vi "运维调试_总磷总氮.vi"() -> ()   [LabVIEW 2016, in "斯坦道总磷总氮.lvlib"]
uses:
  <vilib>/Utility/miscctls.llb/LVPointTypeDef.ctl
  <vilib>/Utility/config.llb/NI_LVConfig.lvlib
  <vilib>/ptbypt/NI_PtbyPt.lvlib
panel:
  in  "总磷参数设置":bool
  in  "总氮参数设置":bool
  in  "模块启用":bool
  in  "串口设置":bool
  in  "备用系数一键写入":bool
  in  "公式一键写入":bool
  in  "流程路径":path=path "C:/Users/std/Documents/斯坦道流程文件/流程.xml"
  in  "曲线模型":cluster{"X^2":dbl, "X":dbl, "B":dbl, "r^2":dbl}(xcontrol)
  out "字符串 2":string
  in  "质控参数设置":bool
  in  "总氮自动测试量程配置":T1
  in  "总磷自动测试量程配置":T1
  out "温度2":sgl
  out "温度1":sgl
  out "ADC":sgl
  out "固件版本号":string
  in  "数组":string[](array[string])
  in  "备用系数写入":bool
  in  "备用系数读取":bool
  in  "备用系数":T2
  in  "量程切换阈值写入":bool
  in  "量程切换阈值读取":bool
  in  "量程切换阈值":cluster{"阈值":dbl, "标液浓度":dbl}
  in  "参数下拉列表":enum16{"总磷", "总氮"}(ring)
  in  "量程下拉列表":enum16{"低量程", "高量程"}(ring)
  in  "测量模式下拉列表":enum16{"水样测量", "零点核查", "跨度核查", "标样核查", "加标回收"}(ring)
  in  "公式":cluster{"X^2":dbl, "X":dbl, "b":dbl}
  in  "写公式":bool
  in  "读公式":bool
  in  "返回":bool
  in  "设置":bool
  out "序列号":string="序列号"
  out "总氮测量数据":T3(xcontrol)
  out "总磷测量数据":T3(xcontrol)
  out "集成报警信息":string
  out "定时启动":bool
  out "总磷总氮运行状态":T4(xcontrol)
  in  "停止":bool
  in  "手动启动":bool
  in  "单步测试":bool
  in  "总磷氨氮调试":u16[](xcontrol)
  out "F3":sgl format="%#.6f"
  out "F2":sgl format="%#.6f"
  out "F1":sgl format="%#.6f"
  out "F0":sgl format="%#.6f"
  out "多列列表框":i32(listbox)
  # "参数设置"
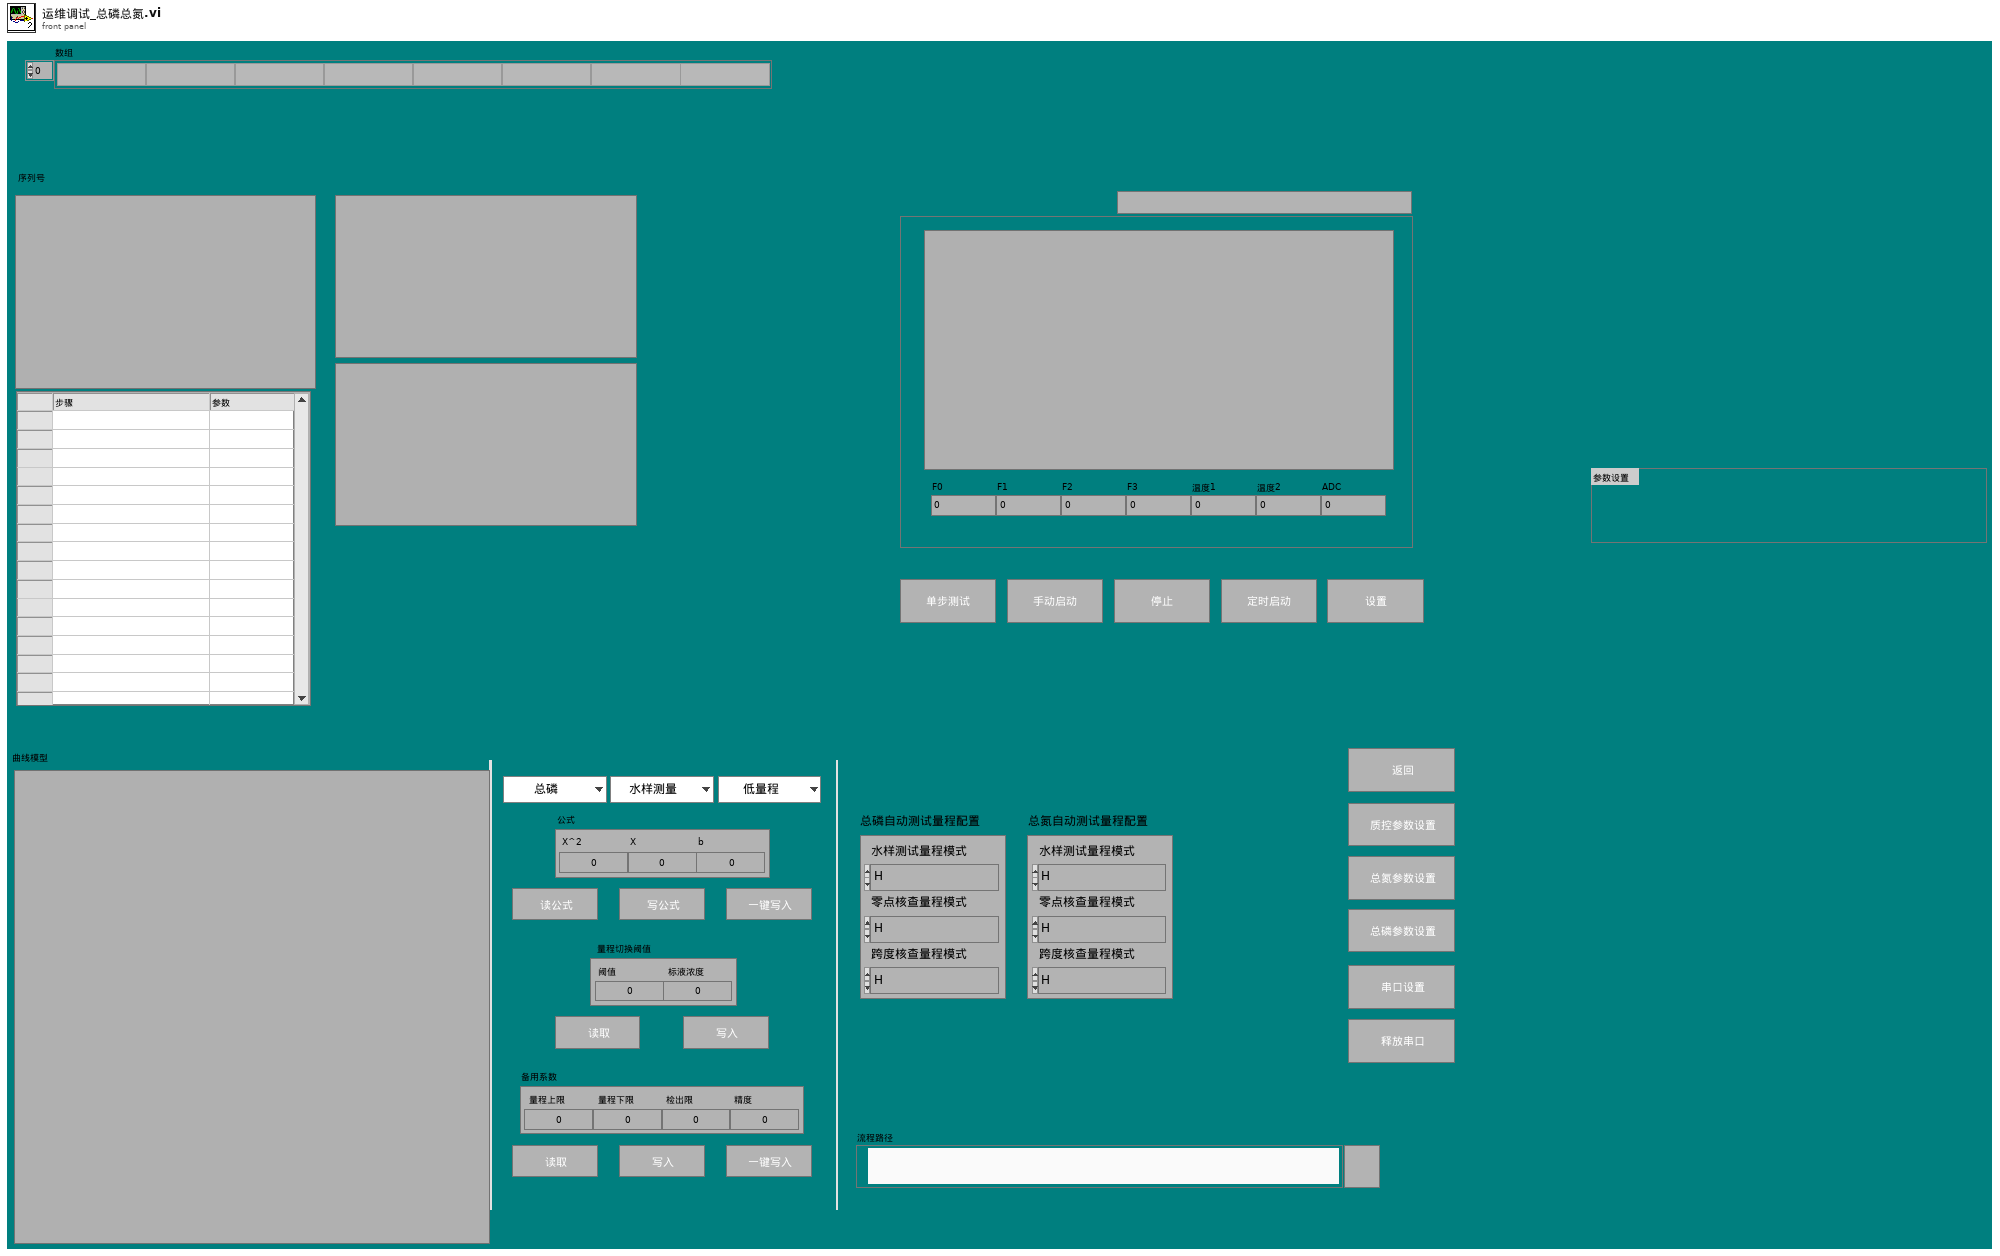
[diagram p1: front panel]
types:
  T1 = cluster{"水样测试量程模式":enum16{"H", "L", "AUTO"}, "空白核查量程模式":enum16{"H", "L", "AUTO"}, "跨度核查量程模式":enum16{"H", "L", "AUTO"}}
  T2 = cluster{"量程上限":dbl, "量程下限":dbl, "检出限":dbl, "精度":dbl}
  T3 = cluster{"flowid":u16, "测量精度":u16, "测量数据区":cluster{"因子编码":u32, "单位":u16, "标样参考值":sgl, "水样数据时间":timestamp, "水样实测值":sgl, "水样数据标识":string, "标样数据时间":timestamp, "标样实测值":sgl, "标样数据标识":string, "空白数据时间":timestamp, "空白实测值":sgl, "空白数据标识":string, "零点核查数据时间":timestamp, "零点核查实测值":sgl, "零点核查数据标识":string, "跨度核查数据时间":timestamp, "跨度核查实测值":sgl, "跨度核查数据标识":string, "加标回收数据时间":timestamp, "加标回收实测值":sgl, "加标回收数据标识":string, "平行样数据时间":timestamp, "平行样实测值":sgl, "平行样数据标识":string, "F0":sgl, "F1":sgl, "F2":sgl, "F3":sgl, "F4":sgl, "F5":sgl, "F6":sgl, "F7":sgl, "温度":sgl, "湿度":sgl, "X值":sgl}}
  T4 = cluster{"系统时间":timestamp, "工作状态":enum16{"空闲", "水样测试", "标样核查", "零点核查", "跨度核查", "空白测试", "平行样测试", "加标回收", "空白校准", "标样校准", "初始化（清洗）"}, "测量模式":enum16{"待机", "连续模式", "周期模式", "定点模式", "受控模式", "手动模式"}, "告警代码":u16, "故障代码":u16, "日志代码":u16, "软件版本":u16, "F0":sgl, "F1":sgl, "F2":sgl, "F3":sgl, "T":sgl, "H":sgl, "id":u16, "flowid":u16, "量程":u16, "总磷控温温度1":sgl, "营养盐控温温度2":sgl, "ADC":sgl}
  T5 = enum16{"启动测量", "标样核查", "零点核查", "跨度核查", "空白测试", "平行样测试", "加标回收", "空白校准", "标样校准", "初始化（清洗）", "停止测试", "仪器重启", "校时", "模式设置", "测量间隔设置"}
  T6 = cluster{"仪器测试类型":enum16{"启动测量", "标样核查", "零点核查", "跨度核查", "空白测试", "平行样测试", "加标回收", "空白校准", "标样校准", "初始化（清洗）", "停止测试", "仪器重启", "校时", "模式设置", "测量间隔设置"}, "周期设置类型":enum16{"定点启动", "间隔启动"}, "定时功能启用":bool, "定时间隔":dbl, "24H周期设置":bool[], "零点核查时间":u16, "跨度核查时间":u16, "质控频次":enum16{"关闭", "每天", "星期一", "星期二", "星期三", "星期四", "星期五", "星期六", "星期日"}}
  T7 = enum16{"关闭", "每天", "星期一", "星期二", "星期三", "星期四", "星期五", "星期六", "星期日"}
  T8 = enum32{"Bad", "Idle", "Run top level", "Running"}
  T9 = typedef "LVDateTimeRec.ctl" = cluster{"秒数的小数部分":dbl, "秒":i32, "分":i32, "时":i32, "日":i32, "月":i32, "年":i32, "天数（周）":i32, "天数（年）":i32, "DST":i32}
  T10 = typedef "LVPointTypeDef.ctl" = cluster{"Horizontal":i16, "Vertical":i16}
  T11 = cluster{"因子编码":u32, "单位":u16, "标样参考值":sgl, "水样数据时间":timestamp, "水样实测值":sgl, "水样数据标识":string, "标样数据时间":timestamp, "标样实测值":sgl, "标样数据标识":string, "空白数据时间":timestamp, "空白实测值":sgl, "空白数据标识":string, "零点核查数据时间":timestamp, "零点核查实测值":sgl, "零点核查数据标识":string, "跨度核查数据时间":timestamp, "跨度核查实测值":sgl, "跨度核查数据标识":string, "加标回收数据时间":timestamp, "加标回收实测值":sgl, "加标回收数据标识":string, "平行样数据时间":timestamp, "平行样实测值":sgl, "平行样数据标识":string, "F0":sgl, "F1":sgl, "F2":sgl, "F3":sgl, "F4":sgl, "F5":sgl, "F6":sgl, "F7":sgl, "温度":sgl, "湿度":sgl, "X值":sgl}
  T12 = enum16{"空闲", "水样测试", "标样核查", "零点核查", "跨度核查", "空白测试", "平行样测试", "加标回收", "空白校准", "标样校准", "初始化（清洗）"}
  T13 = typedef "NI_LVConfig.lvlib/Config Data RefNum.ctl" = refnum<k1>
  T14 = cluster{"启动模式":enum16{"跨度核查", "水样测量", "空白核查", "标样核查", "加标回收"}, "启动参数":u16, "量程":enum16{"低量程", "高量程"}}
  T15 = cluster{"时间标识":timestamp, "设备":string, "日志信息":string, "流程参数":string}
  T16 = cluster{"时间标识":timestamp, "设备":string, "日志信息":string}
  T17 = typedef "LVRowAndColumnUnsignedTypeDef.ctl" = cluster{"Row":u32, "Column":u32}
  T18 = cluster{"参数下拉列表":enum16{"总磷", "总氮"}, "测量模式下拉列表":enum16{"水样测量", "零点核查", "跨度核查", "标样核查", "加标回收"}, "量程下拉列表":enum16{"低量程", "高量程"}}
  T19 = cluster{"站号":u16, "量程切换":enum32{"H", "L", "AUTO"}, "控制命令":enum16{"启动测量", "标样核查", "零点核查", "跨度核查", "空白测试", "平行样测试", "加标回收", "空白校准", "标样校准", "初始化（清洗）", "停止测试", "仪器重启", "校时", "模式设置", "测量间隔设置"}, "模式设置":enum16{"待机", "连续模式", "周期模式", "定点模式", "受控模式", "手动模式"}, "测量间隔":u16}
  T20 = cluster{"总磷跨度值":dbl, "总磷零点标准液浓度":dbl, "总磷跨度标准液浓度":dbl, "总磷标准液标准浓度":dbl, "总氮跨度值":dbl, "总氮零点标准液浓度":dbl, "总氮跨度标准液浓度":dbl, "总氮标准液标准浓度":dbl}
  T21 = cluster{"确定":bool, "总磷跨度值":dbl, "总磷零点标准液浓度":dbl, "总磷跨度标准液浓度":dbl, "总磷标准液标准浓度":dbl, "总氮跨度值":dbl, "总氮零点标准液浓度":dbl, "总氮跨度标准液浓度":dbl, "总氮标准液标准浓度":dbl}
  T22 = cluster{"测量量程":dbl, "测量精度":dbl, "测量间隔":dbl, "消解温度":dbl, "消解时长":dbl, "空白校准时间":timestamp, "曲线截距":dbl, "曲线斜率":dbl, "测量检出限":dbl, "测量信号值":dbl, "线性相关系数":dbl, "二次多项式系数":dbl, "标样校准时间":timestamp, "稀释倍数":dbl, "三项式系数":dbl, "空白标定系数":dbl, "量程系数":dbl, "F0/ORPA":dbl, "F1/ORPB":dbl, "F2/ORPK":dbl, "F3":dbl, "F4":dbl, "F5":dbl, "F6":dbl, "F7":dbl, "X0/滴定数":dbl, "量程":dbl}
  T23 = cluster{"确定":bool, "测量量程":dbl, "测量精度":dbl, "测量间隔":dbl, "消解温度":dbl, "消解时长":dbl, "空白校准时间":timestamp, "曲线截距":dbl, "曲线斜率":dbl, "测量检出限":dbl, "测量信号值":dbl, "线性相关系数":dbl, "二次多项式系数":dbl, "标样校准时间":timestamp, "稀释倍数":dbl, "三项式系数":dbl, "空白标定系数":dbl, "量程系数":dbl, "F0/ORPA":dbl, "F1/ORPB":dbl, "F2/ORPK":dbl, "F3":dbl, "F4":dbl, "F5":dbl, "F6":dbl, "F7":dbl, "X0/滴定数":dbl, "量程":dbl}
  T24 = cluster{"控制命令":enum16{"启动测量", "标样核查", "零点核查", "跨度核查", "空白测试", "平行样测试", "加标回收", "空白校准", "标样校准", "初始化（清洗）", "停止测试", "仪器重启", "校时", "模式设置", "测量间隔设置"}, "周期设置类型":enum16{"定点启动", "间隔启动"}, "定时功能启用":bool, "定时间隔":dbl, "24H周期设置":bool[], "空白核查时间":u16, "跨度核查时间":u16, "质控频次":enum16{"关闭", "每天", "星期一", "星期二", "星期三", "星期四", "星期五", "星期六", "星期日"}}
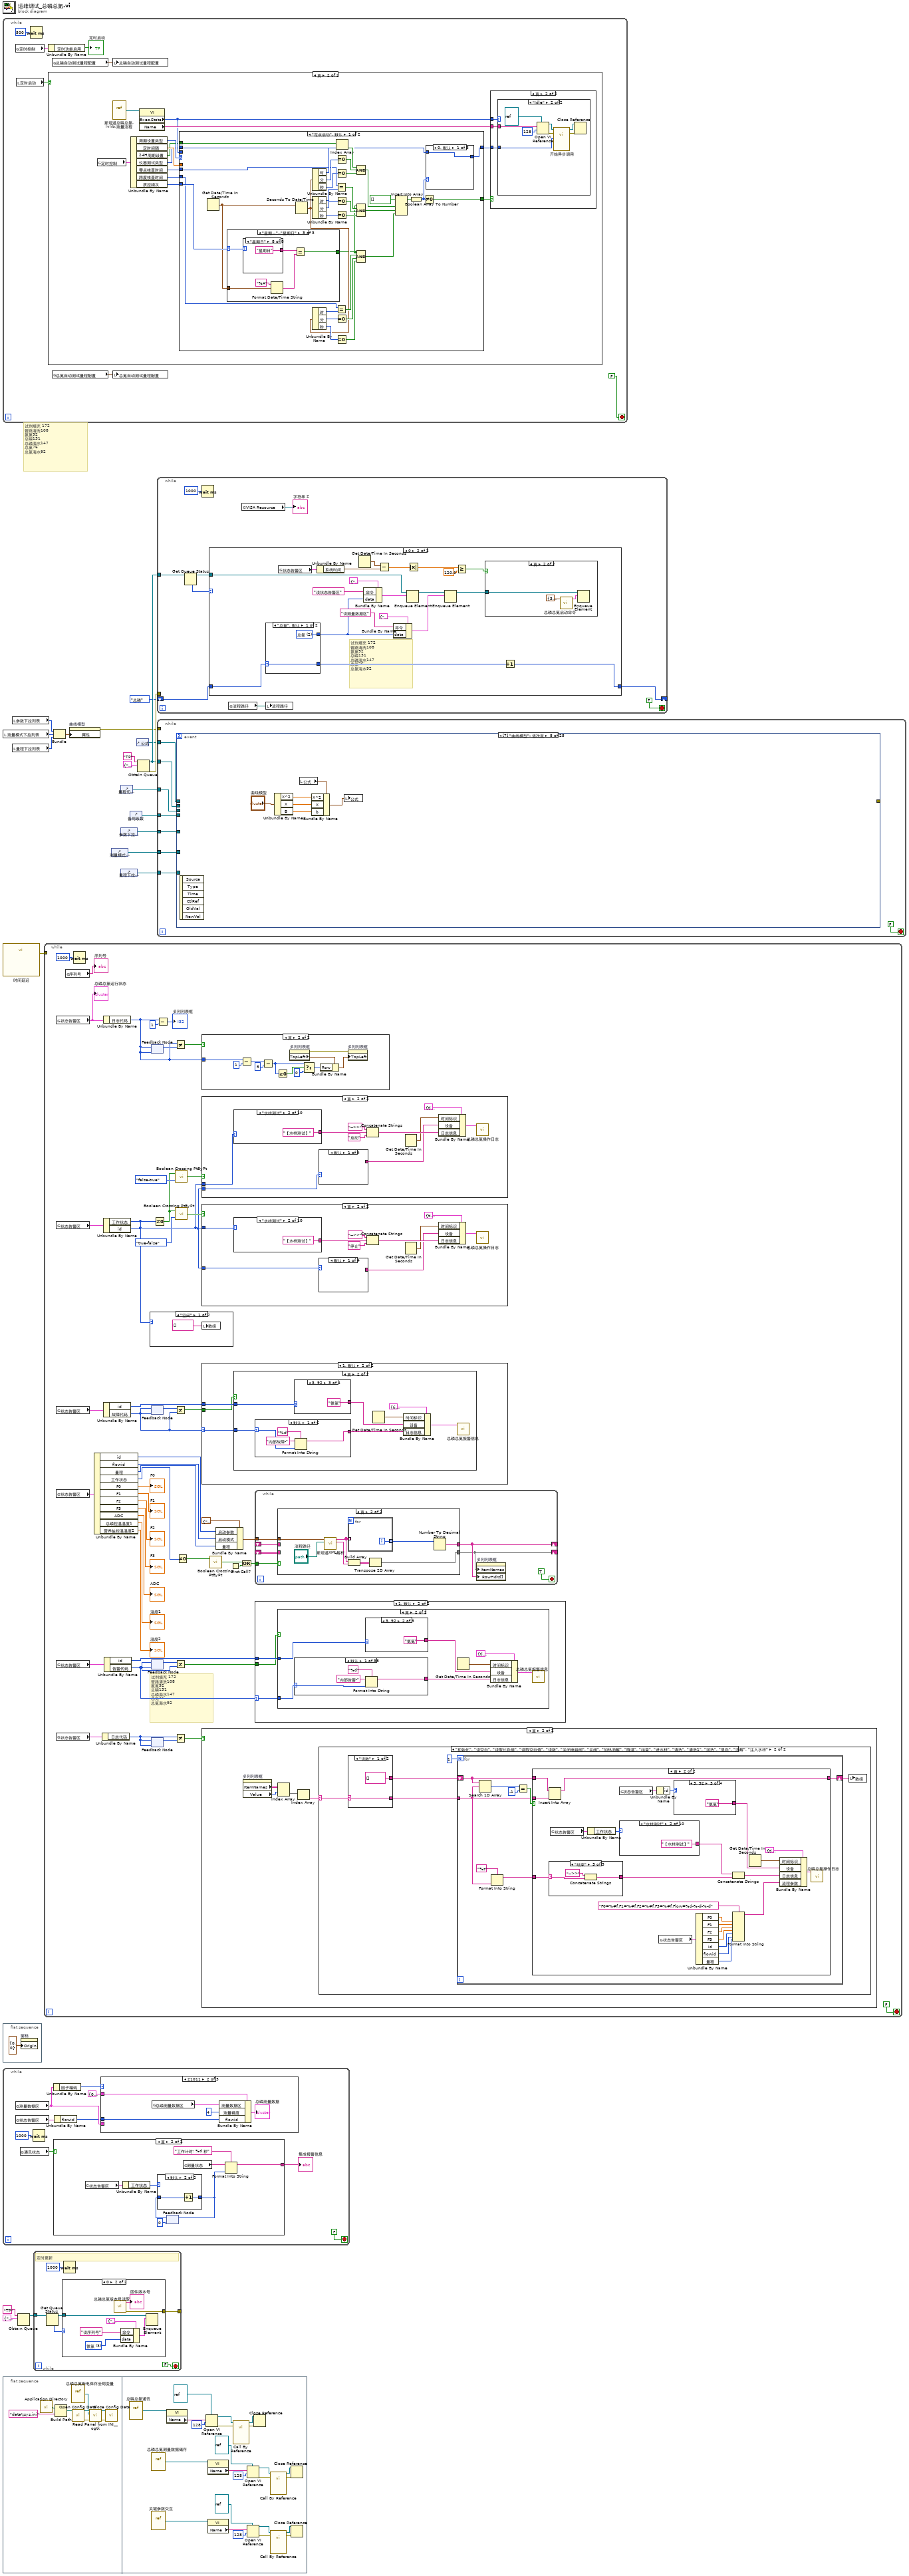
[diagram p0: block diagram]
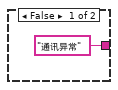
[diagram p3: hidden frame]
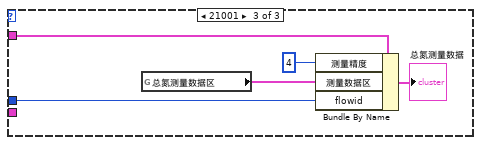
[diagram p6: hidden frame]
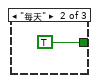
[diagram p9: hidden frame]
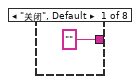
[diagram p10: hidden frame]
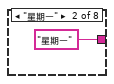
[diagram p11: hidden frame]
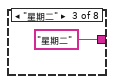
[diagram p12: hidden frame]
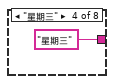
[diagram p13: hidden frame]
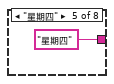
[diagram p14: hidden frame]
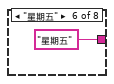
[diagram p15: hidden frame]
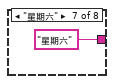
[diagram p16: hidden frame]
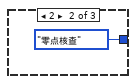
[diagram p17: hidden frame]
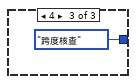
[diagram p18: hidden frame]
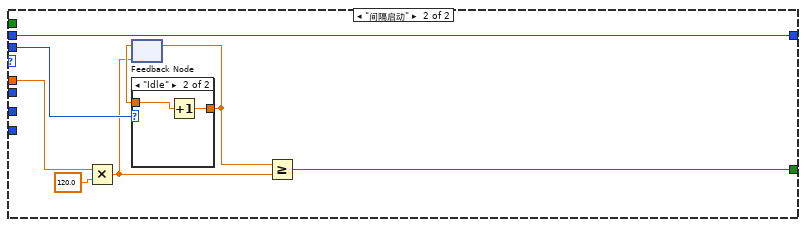
[diagram p19: hidden frame]
diagram:
  # "试剂填充 172 \n管路清洗108\n氨氮92\n总磷131\n总磷海水147\n总氮76\n总氮海水92"
  n1 = while {
    stop <- FALSE stop-if-true
    n2 = global read "总磷总氮断电保存全局变量.vi" "定时控制"() -> (w22:T6)
    n3 = local read "定时启动"() -> (w25:bool)
    n4 = Wait (ms)(milliseconds to wait=u32 500 ("等待时间（毫秒）")) -> ()  [unwired: 1 out]
    n5 = Unbundle By Name(w22) -> ("定时功能启用"=→"定时启动":bool)
    n6 = case shown="真" w25 {
      frame False {
      }
      frame True {
        n7 = global read "总磷总氮断电保存全局变量.vi" "定时控制"() -> (w40:T6)
        n8 = vi-ref "斯坦道总磷总氮.lvlib:测量流程.vi"() -> (w39:refnum<vi>)
        n9 = Unbundle By Name(w40) -> ("周期设置类型"=w37:enum16{"定点启动", "间隔启动"}, "定时间隔"=w35:dbl, "24H周期设置"=w34:bool[], "仪器测试类型"=w33:T5, "零点核查时间"=w32:u16, "跨度核查时间"=w31:u16, "质控频次"=w30:T7)
        n10 = property class="VI"(reference=w39) -> ("Exec.State"=w36:T8, "Name"=w38:string)  [unwired: 1 in, 2 out]
        n11 = case shown="\"定点启动\", 默认" w37 {
          tunnel: w35 -> [_ w97]
          tunnel: w34 -> [w65 _]
          tunnel: w36 -> [_ w100]
          tunnel: [w43 w95] -> w28
          tunnel: w33 -> [w41 w93]
          tunnel: [w69 w93] -> w29
          tunnel: w30 -> [w68 _]
          tunnel: w32 -> [w61 _]
          tunnel: w31 -> [w50 _]
          frame "定点启动", Default {
            n12 = Get Date/Time In Seconds() -> (seconds since 1Jan1904=w67:timestamp)
            n13 = case shown="\"星期一\"..\"星期日\"" w68 {
              selector: w68 -> [_ _ w79]
              tunnel: w67 -> [_ _ w80]
              tunnel: [_ TRUE w76] -> w49
              frame "关闭", Default {
              }
              frame "每天" {
              }
              frame "星期一".."星期日" {
                n14 = case shown="\"星期日\"" w79 {
                  tunnel: ["" ("时间格式字符串(%c)") "星期一" ("时间格式字符串(%c)") "星期二" ("时间格式字符串(%c)") "星期三" ("时间格式字符串(%c)") "星期四" ("时间格式字符串(%c)") "星期五" ("时间格式字符串(%c)") "星期六" ("时间格式字符串(%c)") "星期日" ("时间格式字符串(%c)")] -> w78
                  frame "关闭", Default {
                  }
                  frame "星期一" {
                  }
                  frame "星期二" {
                  }
                  frame "星期三" {
                  }
                  frame "星期四" {
                  }
                  frame "星期五" {
                  }
                  frame "星期六" {
                  }
                  frame "星期日" {
                  }
                }
                n15 = Format Date/Time String(time format string (%c)="%A" ("时间格式字符串(%c)"), seconds (now)=w80) -> (date/time string=w77:string)  [unwired: 1 in]
                n16 = Equal?(x=w78, y=w77) -> (x = y?=w76:bool)
              }
            }
            n17 = Seconds To Date/Time(time stamp (now)=w67) -> (date time rec=w51:T9)  [unwired: 1 in]
            n18 = Unbundle By Name(w51) -> ("时"=w74:i32, "分"=w72:i32, "秒"=w73:i32)
            n19 = Unbundle By Name(w51) -> ("时"=w62:i32, "分"=w64:i32, "秒"=w63:i32)
            n20 = Unbundle By Name(w51) -> ("时"=w54:i32, "分"=w52:i32, "秒"=w53:i32)
            n21 = Equal?(x=w61, y=w62) -> (x = y?=w60:bool)
            n22 = Equal?(x=w50, y=w54) -> (x = y?=w55:bool)
            n23 = Equal To 0?(x=w72) -> (x = 0?=w71:bool)
            n24 = Equal To 0?(x=w73) -> (x = 0?=w70:bool)
            n25 = Equal To 0?(x=w64) -> (x = 0?=w59:bool)
            n26 = Equal To 0?(x=w63) -> (x = 0?=w58:bool)
            n27 = Equal To 0?(x=w52) -> (x = 0?=w56:bool)
            n28 = Equal To 0?(x=w53) -> (x = 0?=w57:bool)
            n29 = Index Array(array=w65, index=w74) -> (element=w66:bool)
            n30 = Compound Arithmetic op=AND ("复合运算")(w66, w71, w70) -> (w47:bool)
            n31 = Compound Arithmetic op=AND ("复合运算")(w49, w60, w59, w58) -> (w46:bool)
            n32 = Compound Arithmetic op=AND ("复合运算")(w49, w55, w56, w57) -> (w45:bool)
            n33 = Insert Into Array(array=bool[] [], new element #1=w47, new element #2=w46, new element #3=w45) -> (w44:bool[])  [unwired: 1 in]
            n34 = Boolean Array To Number(Boolean array=w44) -> (number=w42:u32)
            n35 = Not Equal To 0?(x=w42) -> (x != 0?=w43:bool)
            n36 = case shown="0, 默认" w42 {
              tunnel: [w90 T5."零点核查" ("控制命令") T5."跨度核查" ("控制命令")] -> w69
              tunnel: w41 -> [w90 _ _]
              frame 0, Default {
              }
              frame 2 {
              }
              frame 4 {
              }
            }
          }
          frame "间隔启动" {
            n37 = Multiply(x=w97, y=120.0) -> (x*y=w94:dbl)
            n38 = feedback #1(w94) -> (w99:dbl)
            n39 = case shown="\"Idle\"" w100 {
              tunnel: w99 -> [_ w102]
              tunnel: [_ w101] -> w98
              frame "Bad", Default {
              }
              frame "Idle" {
                n40 = Increment(x=w102) -> (x+1=w101:dbl)
              }
            }
            n41 = feedback-in #1(w98) -> ()
            n42 = Greater Or Equal?(x=w98, y=w94) -> (x >= y?=w95:bool)
          }
        }
        n43 = case shown="真" w28 {
          tunnel: w38 -> [_ w105]
          tunnel: w29 -> [_ w104]
          tunnel: w36 -> [_ w103]
          frame False {
          }
          frame True {
            n44 = case shown="\"Idle\"" w103 {
              tunnel: w105 -> [_ w109]
              tunnel: w104 -> [_ w106]
              frame "Bad", Default {
              }
              frame "Idle" {
                n45 = Open VI Reference(type specifier VI Refnum (for type only)=refnum<vi> refnum, vi path=w109, options=128 ("选项")) -> (vi reference=w110:refnum<vi>, error out=w111:errorcluster)  [unwired: 3 in]
                n46 = call-by-ref "开始异步调用"(reference=w110, error in=w111, "控制命令"=w106) -> (reference out=w112:refnum<vi>, error out=w113:errorcluster)  [unwired: 11 in]
                n47 = Close Reference(reference=w112, error in (no error)=w113) -> ()  [unwired: 1 out]
              }
            }
          }
        }
      }
    }
    n48 = global read "总磷总氮断电保存全局变量.vi" "总磷自动测试量程配置"() -> (w23:T1)
    n49 = global read "总磷总氮断电保存全局变量.vi" "总氮自动测试量程配置"() -> (w24:T1)
    n50 = local write "总磷自动测试量程配置"(w23) -> ()
    n51 = local write "总氮自动测试量程配置"(w24) -> ()
  }
  n52 = local read "测量模式下拉列表"() -> (w3:enum16{"水样测量", "零点核查", "跨度核查", "标样核查", "加标回收"})
  n53 = call "时间延迟"() -> ("error out"=w9:errorcluster)  [unwired: 11 in]
  n54 = flat-sequence {
    frame #0 {
      n55 = property on="窗格" class="Pane"("Origin"=T10 {"Horizontal"=0, "Vertical"=0} ("原点")) -> ()  [unwired: 2 in, 2 out]
    }
  }
  n56 = while {
    stop <- FALSE stop-if-true
    n57 = global read "VAR总磷总氮全局变量.vi" "测量数据区"() -> (w121:T11)
    n58 = global read "VAR总磷总氮全局变量.vi" "状态告警区"() -> (w117:T4)
    n59 = global read "VAR总磷总氮全局变量.vi" "通讯状态"() -> (w119:bool)
    n60 = Wait (ms)(milliseconds to wait=u32 1000 ("等待时间（毫秒）")) -> ()  [unwired: 1 out]
    n61 = Unbundle By Name(w121) -> ("因子编码"=w120:u32)
    n62 = case shown="真" w119 {
      tunnel: ["通讯异常" ("集成报警信息") w126] -> w118
      frame False {
      }
      frame True {
        n63 = global read "VAR总磷总氮全局变量.vi" "状态告警区"() -> (w132:T4)
        n64 = Unbundle By Name(w132) -> ("工作状态"=w131:T12)
        n65 = feedback #2(0) -> (w129:i32)
        n66 = case shown="默认" w131 {
          tunnel: w129 -> [_ w134]
          tunnel: [_ w133] -> w127
          frame "空闲" {
          }
          frame Default {
            n67 = Increment(x=w134) -> (x+1=w133:i32)
          }
        }
        n68 = feedback-in #2(w127) -> ()
        n69 = global read "VAR总磷总氮全局变量.vi" "测量状态"() -> (w125:string)
        n70 = Format Into String(format string="工作计时: %d 秒" ("格式字符串"), initial string=w125, w127) -> (resulting string=w126:string)  [unwired: 1 in, 1 out]
      }
    }
    "集成报警信息" <- w118
    n71 = Unbundle By Name(w117) -> ("flowid"=w116:u16)
    n72 = case shown="21011" w120 {
      tunnel: w121 -> [_ _ _]
      tunnel: w116 -> [_ w137 w143]
      tunnel: T3 {"flowid"=0, "测量精度"=0, "测量数据区"={"因子编码"=0, "单位"=0, "标样参考值"=0.0, "水样数据时间"=timestamp(0 s since 1904-01-01), "水样实测值"=0.0, "水样数据标识"="", "标样数据时间"=timestamp(0 s since 1904-01-01), "标样实测值"=0.0, "标样数据标识"="", "空白数据时间"=timestamp(0 s since 1904-01-01), "空白实测值"=0.0, "空白数据标识"="", "零点核查数据时间"=timestamp(0 s since 1904-01-01), "零点核查实测值"=0.0, "零点核查数据标识"="", "跨度核查数据时间"=timestamp(0 s since 1904-01-01), "跨度核查实测值"=0.0, "跨度核查数据标识"="", "加标回收数据时间"=timestamp(0 s since 1904-01-01), "加标回收实测值"=0.0, "加标回收数据标识"="", "平行样数据时间"=timestamp(0 s since 1904-01-01), "平行样实测值"=0.0, "平行样数据标识"="", "F0"=0.0, "F1"=0.0, "F2"=0.0, "F3"=0.0, "F4"=0.0, "F5"=0.0, "F6"=0.0, "F7"=0.0, "温度"=0.0, "湿度"=0.0, "X值"=0.0}} ("总氮测量数据") -> [_ w136 w142]
      frame Default {
      }
      frame 21011 {
        n73 = global read "VAR总磷总氮全局变量.vi" "总磷测量数据区"() -> (w135:T11)
        n74 = Bundle By Name(cluster=w136, "测量数据区"=w135, "测量精度"=u16 4, "flowid"=w137) -> (→"总磷测量数据":T3)
      }
      frame 21001 {
        n75 = global read "VAR总磷总氮全局变量.vi" "总氮测量数据区"() -> (w140:T11)
        n76 = Bundle By Name(cluster=w142, "测量精度"=u16 4, "测量数据区"=w140, "flowid"=w143) -> (→"总氮测量数据":T3)
      }
    }
  }
  n77 = flat-sequence {
    frame #0 {
      n78 = call <vilib>:"Application Directory.vi"() -> ("Application Directory"=w152:path)
      n79 = Build Path(base path=w152, name or relative path="data\\sys.ini" ("名称或相对路径")) -> (appended path=w150:path)
      n80 = vi-ref "总磷总氮断电保存全局变量.vi"() -> (w148:refnum<vi>)
      n81 = call <vilib>:"Open Config Data.vi"("configuration file path"=w150) -> ("error out"=w146:errorcluster, "refnum"=w149:T13)  [unwired: 8 in, 1 out]
      n82 = call <userlib>:"Read Panel from INI__ogtk.vi"("error in (no error)"=w146, "VI ref"=w148, "refnum"=w149) -> ("error out"=w145:errorcluster, "refnum out"=w147:T13)  [unwired: 7 in]
      n83 = call <vilib>:"Close Config Data.vi"("error in (no error)"=w145, "refnum"=w147) -> ()  [unwired: 8 in, 2 out]
    }
    frame #1 {
      n84 = vi-ref "总磷总氮通讯.vi"() -> (w176:refnum<vi>)
      n85 = vi-ref "总磷总氮测量数据储存.vi"() -> (w168:refnum<vi>)
      n86 = vi-ref "关键参数交互.vi"() -> (w153:refnum<vi>)
      n87 = property class="VI"(reference=w176) -> ("Name"=w175:string)  [unwired: 1 in, 2 out]
      n88 = Open VI Reference(type specifier VI Refnum (for type only)=refnum<vi> refnum, vi path=w175, options=128 ("选项")) -> (vi reference=w173:refnum<vi>, error out=w171:errorcluster)  [unwired: 3 in]
      n89 = property class="VI"(reference=w168) -> ("Name"=w161:string)  [unwired: 1 in, 2 out]
      n90 = property class="VI"(reference=w153) -> ("Name"=w160:string)  [unwired: 1 in, 2 out]
      n91 = call-by-ref "?"(reference=w173, error in=w171) -> (reference out=w169:refnum<vi>, error out=w170:errorcluster)  [unwired: 12 in]
      n92 = Open VI Reference(type specifier VI Refnum (for type only)=refnum<vi> refnum, vi path=w161, options=128 ("选项")) -> (vi reference=w163:refnum<vi>, error out=w165:errorcluster)  [unwired: 3 in]
      n93 = Open VI Reference(type specifier VI Refnum (for type only)=refnum<vi> refnum, vi path=w160, options=128 ("选项")) -> (vi reference=w158:refnum<vi>, error out=w156:errorcluster)  [unwired: 3 in]
      n94 = Close Reference(reference=w169, error in (no error)=w170) -> ()  [unwired: 1 out]
      n95 = call-by-ref "?"(reference=w163, error in=w165) -> (reference out=w167:refnum<vi>, error out=w166:errorcluster)  [unwired: 12 in]
      n96 = call-by-ref "?"(reference=w158, error in=w156) -> (reference out=w154:refnum<vi>, error out=w155:errorcluster)  [unwired: 12 in]
      n97 = Close Reference(reference=w167, error in (no error)=w166) -> ()  [unwired: 1 out]
      n98 = Close Reference(reference=w154, error in (no error)=w155) -> ()  [unwired: 1 out]
    }
  }
  n99 = local read "参数下拉列表"() -> (w2:enum16{"总磷", "总氮"})
  n100 = local read "量程下拉列表"() -> (w1:enum16{"低量程", "高量程"})
  n101 = Obtain Queue(name (unnamed)="TP" ("名称（未命名）"), element data type=cluster{"命令":string, "data":variant} {"命令"="", "data"=variant}) -> (queue out=w6:refnum<queue>)  [unwired: 3 in, 2 out]
  n102 = while {
    tunnel: w6 -> [w181]
    tunnel: [w179] -> _
    stop <- FALSE stop-if-true
    # "定时更新"
    n103 = Get Queue Status(queue=w181) -> (queue out=w178:refnum<queue>, # elements in queue=w177:i32)  [unwired: 2 in, 6 out]
    n104 = case shown="0" w177 {
      tunnel: w178 -> [_ w186]
      tunnel: [_ w183] -> w179
      frame Default {
      }
      frame 0 {
        w187 = u16 3 items=["总磷"=1, "氨氮"=3] ("站号")
        n105 = call "总磷总氮版本号读取.vi"() -> ("error out"=w183:errorcluster, "固件版本号"=→"固件版本号":string)  [unwired: 10 in]
        n106 = Bundle By Name(cluster=cluster{"命令":string, "data":variant} {"命令"="", "data"=variant} ("元素"), "命令"="读序列号", "data"=w187) -> (w185:cluster{"命令":string, "data":variant})
        n107 = Enqueue Element(queue=w186, element=w185) -> ()  [unwired: 2 in, 3 out]
      }
    }
    n108 = Wait (ms)(milliseconds to wait=u32 1000 ("等待时间（毫秒）")) -> ()  [unwired: 1 out]
  }
  n109 = while {
    tunnel: w9 -> [_]
    stop <- FALSE stop-if-true
    # "试剂填充 172 \n管路清洗108\n氨氮92\n总磷131\n总磷海水147\n总氮76\n总氮海水92"
    n110 = global read "VAR总磷总氮全局变量.vi" "状态告警区"() -> (w223:T4)
    "总磷总氮运行状态" <- w223
    n111 = global read "VAR总磷总氮全局变量.vi" "状态告警区"() -> (w210:T4)
    n112 = global read "VAR总磷总氮全局变量.vi" "状态告警区"() -> (w215:T4)
    n113 = global read "VAR总磷总氮全局变量.vi" "状态告警区"() -> (w231:T4)
    n114 = global read "VAR总磷总氮全局变量.vi" "状态告警区"() -> (w220:T4)
    n115 = global read "VAR总磷总氮全局变量.vi" "状态告警区"() -> (w208:T4)
    n116 = global read "VAR总磷总氮全局变量.vi" "序列号"() -> (→"序列号":string)
    n117 = Wait (ms)(milliseconds to wait=u32 1000 ("等待时间（毫秒）")) -> ()  [unwired: 1 out]
    n118 = Unbundle By Name(w231) -> ("id"=w228:u16, "flowid"=w230:u16, "量程"=w229:u16, "工作状态"=w198:T12, "F0"=→"F0":sgl, "F1"=→"F1":sgl, "F2"=→"F2":sgl, "F3"=→"F3":sgl, "ADC"=→"ADC":sgl, "总磷控温温度1"=→"温度1":sgl, "营养盐控温温度2"=→"温度2":sgl)
    n119 = Unbundle By Name(w208) -> ("日志代码"=w207:u16)
    n120 = Unbundle By Name(w223) -> ("日志代码"=w204:u16)
    n121 = Unbundle By Name(w210) -> ("工作状态"=w191:T12, "id"=w190:u16)
    n122 = Unbundle By Name(w215) -> ("id"=w214:u16, "故障代码"=w211:u16)
    n123 = Unbundle By Name(w220) -> ("id"=w219:u16, "告警代码"=w216:u16)
    n124 = case shown="\"空闲\"" w191 {
      frame "空闲" {
        n125 = local write "数组"(string[] [] ("数组")) -> ()
      }
      frame "水样测试", Default {
      }
    }
    n126 = feedback-in #3(w204) -> ()
    n127 = feedback #3(w204) -> (w236:u16)
    n128 = feedback #4(w211) -> (w212:u16)
    n129 = feedback-in #4(w211) -> ()
    n130 = feedback #5(w216) -> (w217:u16)
    n131 = feedback-in #5(w216) -> ()
    n132 = feedback #6(w207) -> (w209:u16)
    n133 = feedback-in #6(w207) -> ()
    n134 = Not Equal To 0?(x=w191) -> (x != 0?=w193:bool)
    n135 = Subtract(x=w204, y=1) -> (x-y=→"多列列表框":i32)
    n136 = Not Equal?(x=w204, y=w236) -> (x != y?=w235:bool)
    n137 = Not Equal?(x=w212, y=w211) -> (x != y?=w213:bool)
    n138 = Not Equal?(x=w217, y=w216) -> (x != y?=w218:bool)
    n139 = Not Equal?(x=w207, y=w209) -> (x != y?=w206:bool)
    n140 = call <vilib>:"Boolean Crossing PtByPt.vi"("direction"=enum16{"either", "false-true", "true-false"}."false-true", "input"=w193) -> ("crossing"=w195:bool)  [unwired: 1 in]
    n141 = call <vilib>:"Boolean Crossing PtByPt.vi"("direction"=enum16{"either", "false-true", "true-false"}."true-false", "input"=w193) -> ("crossing"=w192:bool)  [unwired: 1 in]
    n142 = Not Equal To 0?(x=w198) -> (x != 0?=w233:bool)
    n143 = case shown="真" w235 {
      tunnel: w204 -> [_ w446]
      frame False {
      }
      frame True {
        n144 = Subtract(x=w446, y=1) -> (x-y=w444:i32)
        n145 = Subtract(x=w444, y=5) -> (x-y=w448:i32)
        n146 = Greater Or Equal To 0?(x=w448) -> (x >= 0?=w447:bool)
        n147 = property on="多列列表框" class="MCListbox (严格)"() -> (error out=w452:errorcluster, "TopLeft"=w453:T17)  [unwired: 2 in, 1 out]
        n148 = Select(t=w448, s=w447, f=0) -> (s? t:f=w449:i32)
        n149 = Bundle By Name(cluster=w453, "Row"=w449) -> (w454:T17)
        n150 = property on="多列列表框" class="MCListbox (严格)"(error in=w452, "TopLeft"=w454) -> ()  [unwired: 1 in, 2 out]
      }
    }
    n151 = case shown="真" w195 {
      tunnel: w191 -> [_ w263]
      tunnel: w190 -> [_ w262]
      frame False {
      }
      frame True {
        n152 = case shown="\"水样测试\"" w263 {
          tunnel: [_ "【水样测试】" ("字符串") "【标样核查】" ("字符串") "【零点核查】" ("字符串") "【跨度核查】" ("字符串") "【空白测试】" ("字符串") "【平行样测试】" ("字符串") "【加标回收】" ("字符串") "【空白校准】" ("字符串") "【标样校准】" ("字符串")] -> w270
          frame "空闲", Default {
          }
          frame "水样测试" {
          }
          frame "标样核查" {
          }
          frame "零点核查" {
          }
          frame "跨度核查" {
          }
          frame "空白测试" {
          }
          frame "平行样测试" {
          }
          frame "加标回收" {
          }
          frame "空白校准" {
          }
          frame "标样校准" {
          }
        }
        n153 = case shown="默认" w262 {
          tunnel: [_ "总磷" ("table输入") "氨氮" ("table输入") "总氮" ("table输入")] -> w266
          frame Default {
          }
          frame 1, 131 {
          }
          frame 3, 92 {
          }
          frame 2, 76 {
          }
        }
        n154 = Concatenate Strings("-->>" ("字符串"), w270, "启动" ("字符串")) -> (w269:string)
        n155 = Get Date/Time In Seconds() -> (seconds since 1Jan1904=w267:timestamp)
        n156 = Bundle By Name(cluster=T15 {"时间标识"=timestamp(0 s since 1904-01-01), "设备"="", "日志信息"="", "流程参数"=""} ("data in"), "时间标识"=w267, "设备"=w266, "日志信息"=w269) -> (w261:T15)
        n157 = call "总磷总氮操作日志.vi"("data in"=w261) -> ()  [unwired: 11 in]
      }
    }
    n158 = case shown="真" w192 {
      tunnel: w191 -> [_ w241]
      tunnel: w190 -> [_ w240]
      frame False {
      }
      frame True {
        n159 = case shown="\"水样测试\"" w241 {
          tunnel: [_ "【水样测试】" ("字符串") "【标样核查】" ("字符串") "【零点核查】" ("字符串") "【跨度核查】" ("字符串") "【空白测试】" ("字符串") "【平行样测试】" ("字符串") "【加标回收】" ("字符串") "【空白校准】" ("字符串") "【标样校准】" ("字符串")] -> w248
          frame "空闲", Default {
          }
          frame "水样测试" {
          }
          frame "标样核查" {
          }
          frame "零点核查" {
          }
          frame "跨度核查" {
          }
          frame "空白测试" {
          }
          frame "平行样测试" {
          }
          frame "加标回收" {
          }
          frame "空白校准" {
          }
          frame "标样校准" {
          }
        }
        n160 = case shown="默认" w240 {
          tunnel: [_ "总磷" ("table输入") "氨氮" ("table输入") "总氮" ("table输入")] -> w244
          frame Default {
          }
          frame 1, 131 {
          }
          frame 3, 92 {
          }
          frame 2, 76 {
          }
        }
        n161 = Concatenate Strings("-->>" ("字符串"), w248, "停止" ("字符串")) -> (w247:string)
        n162 = Get Date/Time In Seconds() -> (seconds since 1Jan1904=w245:timestamp)
        n163 = Bundle By Name(cluster=T15 {"时间标识"=timestamp(0 s since 1904-01-01), "设备"="", "日志信息"="", "流程参数"=""} ("data in"), "时间标识"=w245, "设备"=w244, "日志信息"=w247) -> (w239:T15)
        n164 = call "总磷总氮操作日志.vi"("data in"=w239) -> ()  [unwired: 11 in]
      }
    }
    n165 = case shown="1, 默认" w211 {
      selector: w211 -> [_ w351]
      tunnel: w214 -> [_ w352]
      tunnel: w213 -> [_ w350]
      frame 0 {
      }
      frame 1, Default {
        n166 = case shown="真" w350 {
          tunnel: w352 -> [_ w359]
          tunnel: w351 -> [_ w354]
          frame False {
          }
          frame True {
            n167 = case shown="默认" w354 {
              selector: w354 -> [w361 _ _ _ _ _]
              tunnel: [w360 "无故障" "电机故障" "温度故障" "通讯故障" "滴定故障"] -> w353
              frame Default {
                n168 = Format Into String(format string="%d" ("格式字符串"), initial string="内部故障-" ("工作状态"), w361) -> (resulting string=w360:string)  [unwired: 1 in, 1 out]
              }
              frame 0 {
              }
              frame 1 {
              }
              frame 2 {
              }
              frame 3 {
              }
              frame 4 {
              }
            }
            n169 = case shown="3, 92" w359 {
              tunnel: [_ "总磷" ("table输入") "氨氮" ("table输入") "总氮" ("table输入")] -> w355
              frame Default {
              }
              frame 1, 131 {
              }
              frame 3, 92 {
              }
              frame 2, 76 {
              }
            }
            n170 = Get Date/Time In Seconds() -> (seconds since 1Jan1904=w356:timestamp)
            n171 = Bundle By Name(cluster=T16 {"时间标识"=timestamp(0 s since 1904-01-01), "设备"="", "日志信息"=""} ("data in"), "时间标识"=w356, "设备"=w355, "日志信息"=w353) -> (w357:T16)
            n172 = call "总磷总氮报警信息.vi"("data in"=w357) -> ()  [unwired: 10 in, 1 out]
          }
        }
      }
    }
    n173 = case shown="真" w206 {
      frame False {
      }
      frame True {
        n174 = property on="多列列表框" class="MCListbox (严格)"() -> ("ItemNames"=w286:string[][], "Value"=w287:i32)  [unwired: 2 in, 2 out]
        n175 = Index Array(array=w286, index (row)=w287) -> (element=w285:string[])  [unwired: 1 in]
        n176 = Index Array(array=w285) -> (element=w284:string)  [unwired: 1 in]
        n177 = case shown="\"初始化\", \"读空白\", \"读取比色值\", \"读取空白值\", \"读数\", \"关闭电磁阀\", \"关阀\", \"加热消解\", \"降温\", \"结束\", \"进水样\", \"清洗\", \"清洗1\", \"润洗\", \"显色\", \"消解\", \"注入水样\"" w284 {
          selector: w284 -> [_ w290]
          frame Default {
          }
          frame "初始化", "读空白", "读取比色值", "读取空白值", "读数", "关闭电磁阀", "关阀", "加热消解", "降温", "结束", "进水样", "清洗", "清洗1", "润洗", "显色", "消解", "注入水样" {
            n178 = case shown="\"读数\"" w290 {
              selector: w290 -> [w294 w296]
              tunnel: [w294 w296] -> w289
              tunnel: [string[] [] ("数组") "数组"] -> w288
              frame "读数" {
              }
              frame Default {
              }
            }
            n179 = for {
              N: 1 -> [_]
              tunnel: w289 -> [w298]
              shift-right: [w297] -> w291
              shift-left: w288 -> [w299]
              n180 = Search 1D Array(1D array=w299, element=w298) -> (index of element=w302:i32)  [unwired: 1 in]
              n181 = Format Into String(format string="%s" ("格式字符串"), w298) -> (resulting string=w303:string)  [unwired: 2 in, 1 out]
              n182 = Equal?(x=w302, y=-1) -> (x = y?=w300:bool)
              n183 = case shown="真" w300 {
                tunnel: w303 -> [_ w311]
                tunnel: w299 -> [w305 w315]
                tunnel: w298 -> [_ w314]
                tunnel: [w305 w313] -> w297
                frame False {
                }
                frame True {
                  n184 = Insert Into Array(array=w315, new element=w314) -> (w313:string[])  [unwired: 1 in]
                  n185 = case shown="\"结束\"" w311 {
                    selector: w311 -> [w340 w343 w346]
                    tunnel: [w340 w342 w345] -> w310
                    frame Default {
                    }
                    frame "初始化" {
                      n186 = Concatenate Strings("-->>" ("字符串"), w343) -> (w342:string)
                    }
                    frame "结束" {
                      n187 = Concatenate Strings("-->>" ("字符串"), w346) -> (w345:string)
                    }
                  }
                  n188 = global read "VAR总磷总氮全局变量.vi" "状态告警区"() -> (w309:T4)
                  n189 = Unbundle By Name(w309) -> ("工作状态"=w308:T12)
                  n190 = global read "VAR总磷总氮全局变量.vi" "状态告警区"() -> (w330:T4)
                  n191 = case shown="\"水样测试\"" w308 {
                    tunnel: [_ "【水样测试】" ("字符串") "【标样核查】" ("字符串") "【零点核查】" ("字符串") "【跨度核查】" ("字符串") "【空白测试】" ("字符串") "【平行样测试】" ("字符串") "【加标回收】" ("字符串") "【空白校准】" ("字符串") "【标样校准】" ("字符串")] -> w306
                    frame "空闲", Default {
                    }
                    frame "水样测试" {
                    }
                    frame "标样核查" {
                    }
                    frame "零点核查" {
                    }
                    frame "跨度核查" {
                    }
                    frame "空白测试" {
                    }
                    frame "平行样测试" {
                    }
                    frame "加标回收" {
                    }
                    frame "空白校准" {
                    }
                    frame "标样校准" {
                    }
                  }
                  n192 = Unbundle By Name(w330) -> ("id"=w329:u16)
                  n193 = global read "VAR总磷总氮全局变量.vi" "状态告警区"() -> (w325:T4)
                  n194 = case shown="3, 92" w329 {
                    tunnel: [_ "总磷" ("table输入") "氨氮" ("table输入") "总氮" ("table输入")] -> w327
                    frame Default {
                    }
                    frame 1, 131 {
                    }
                    frame 3, 92 {
                    }
                    frame 2, 76 {
                    }
                  }
                  n195 = Unbundle By Name(w325) -> ("F0"=w322:sgl, "F1"=w321:sgl, "F2"=w320:sgl, "F3"=w319:sgl, "id"=w318:u16, "flowid"=w317:u16, "量程"=w316:u16)
                  n196 = Concatenate Strings(w306, w310) -> (w307:string)
                  n197 = Format Into String(format string="F0=%#f,F1=%#f,F2=%#f,F3=%#f,Flow=%d-%-d-%-d" ("格式字符串"), w322, w321, w320, w319, w318, w317, w316) -> (resulting string=w323:string)  [unwired: 2 in, 1 out]
                  n198 = Get Date/Time In Seconds() -> (seconds since 1Jan1904=w326:timestamp)
                  n199 = Bundle By Name(cluster=T15 {"时间标识"=timestamp(0 s since 1904-01-01), "设备"="", "日志信息"="", "流程参数"=""} ("data in"), "时间标识"=w326, "设备"=w327, "日志信息"=w307, "流程参数"=w323) -> (w328:T15)
                  n200 = call "总磷总氮操作日志.vi"("data in"=w328) -> ()  [unwired: 11 in]
                }
              }
            }
            n201 = local write "数组"(w291) -> ()
          }
        }
      }
    }
    n202 = call <vilib>:"Boolean Crossing PtByPt.vi"("input"=w233) -> ("crossing"=w197:bool)  [unwired: 2 in]
    n203 = Bundle By Name(cluster=T14 {"启动模式"=enum."跨度核查", "启动参数"=1, "量程"=enum."低量程"} ("参数簇"), "启动参数"=w228, "启动模式"=w230, "量程"=w229) -> (w222:T14)
    n204 = First Call?() -> (First Call?: T/F=w234:bool)
    n205 = Or(x=w197, y=w234) -> (x .or. y?=w232:bool)
    n206 = while {
      tunnel: w232 -> [w432]
      tunnel: w222 -> [w431]
      shift-right: [w426] -> _
      shift-left: _ -> [w428]
      shift-right: [w427] -> _
      shift-left: _ -> [w429]
      stop <- TRUE stop-if-true
      n207 = case shown="真" w432 {
        tunnel: [w434 w442] -> w427
        tunnel: [w433 w441] -> w426
        tunnel: w431 -> [_ w436]
        tunnel: w429 -> [w434 _]
        tunnel: w428 -> [w433 _]
        frame False {
        }
        frame True {
          n208 = call "斯坦道XML解析.vi"("添加的路径"="流程路径", "参数簇"=w436) -> ("步骤时间"=w437:string[], "步骤名"=w439:string[])  [unwired: 8 in]
          n209 = for {
            tunnel: w439 -> [_] mode=indexing
            tunnel: [w443] -> w440 mode=indexing
            i -> [w443]
          }
          n210 = Build Array(w439, w437) -> (w438:string[][])
          n211 = Transpose 2D Array(2D array=w438) -> (transposed array=w441:string[][])
          n212 = Number To Decimal String(number=w440) -> (decimal integer string=w442:string[])  [unwired: 1 in]
        }
      }
      n213 = property on="多列列表框" class="MCListbox (严格)"("ItemNames"=w426, "RowHdrs[]"=w427) -> ()  [unwired: 2 in, 2 out]
    }
    n214 = case shown="1, 默认" w216 {
      selector: w216 -> [_ w373]
      tunnel: w219 -> [_ w374]
      tunnel: w218 -> [_ w372]
      frame 0 {
      }
      frame 1, Default {
        n215 = case shown="真" w372 {
          tunnel: w374 -> [_ w381]
          tunnel: w373 -> [_ w375]
          frame False {
          }
          frame True {
            n216 = case shown="默认" w375 {
              selector: w375 -> [w383 _ _ _ _ _ _ _ _ _ _ _ _ _ _ _ _ _ _ _ _ _ _ _ _ _ _ _ _ _ _ _ _ _ _ _ _ _]
              tunnel: [w382 "无告警" "缺试剂告警" "缺水样告警" "缺蒸馏水告警" "缺标液告警" "仪表漏液告警" "标定异常告警" "超量程告警" "加热异常" "低试剂预警" "超上限告警" "超下限告警" "仪表内部其他异常" "滴定异常告警" "电极异常告警" "量程切换告警" "参数设置告警" "PH电极电位异常" "电导率电极异常" "浊度光度异常" "溶解氧电极异常" "溶解氧光强异常" "温度异常告警" "PH异常告警" "溶解氧异常告警" "电导率异常告警" "浊度异常告警" "叶绿素异常告警" "藻密度异常告警" "蓝绿藻异常告警" "ORP异常告警" "氨氮异常告警" "清洁刷异常告警" "SD卡异常告警" "蓝牙异常告警" "WiFi异常告警" "流程异常告警"] -> w376
              frame Default {
                n217 = Format Into String(format string="%d" ("格式字符串"), initial string="内部告警-" ("工作状态"), w383) -> (resulting string=w382:string)  [unwired: 1 in, 1 out]
              }
              frame 0 {
              }
              frame 1 {
              }
              frame 2 {
              }
              frame 3 {
              }
              frame 4 {
              }
              frame 5 {
              }
              frame 6 {
              }
              frame 7 {
              }
              frame 8 {
              }
              frame 9 {
              }
              frame 10 {
              }
              frame 11 {
              }
              frame 12 {
              }
              frame 13 {
              }
              frame 14 {
              }
              frame 15 {
              }
              frame 16 {
              }
              frame 17 {
              }
              frame 18 {
              }
              frame 19 {
              }
              frame 20 {
              }
              frame 21 {
              }
              frame 22 {
              }
              frame 23 {
              }
              frame 24 {
              }
              frame 25 {
              }
              frame 26 {
              }
              frame 27 {
              }
              frame 28 {
              }
              frame 29 {
              }
              frame 30 {
              }
              frame 31 {
              }
              frame 32 {
              }
              frame 33 {
              }
              frame 34 {
              }
              frame 35 {
              }
              frame 36 {
              }
            }
            n218 = case shown="3, 92" w381 {
              tunnel: ["总磷" ("table输入") "氨氮" ("table输入") "总氮" ("table输入")] -> w377
              frame 1, 131 {
              }
              frame 3, 92 {
              }
              frame 2, 76, Default {
              }
            }
            n219 = Get Date/Time In Seconds() -> (seconds since 1Jan1904=w378:timestamp)
            n220 = Bundle By Name(cluster=T16 {"时间标识"=timestamp(0 s since 1904-01-01), "设备"="", "日志信息"=""} ("data in"), "时间标识"=w378, "设备"=w377, "日志信息"=w376) -> (w379:T16)
            n221 = call "总磷总氮报警信息.vi"("data in"=w379) -> ()  [unwired: 10 in, 1 out]
          }
        }
      }
    }
  }
  n222 = Bundle("参数下拉列表"=w2, "测量模式下拉列表"=w3, "量程下拉列表"=w1) -> (w4:T18)  [unwired: 1 in]
  n223 = property on="曲线模型" class="曲线模型 (严格)"("属性"=w4) -> (error out=w5:errorcluster)  [unwired: 2 in, 1 out]
  n224 = control-ref of="测量模式下拉列表"() -> (w13:refnum<vi>)
  n225 = control-ref of="量程切换阈值"() -> (w11:refnum<vi>)
  n226 = control-ref of="参数下拉列表"() -> (w14:refnum<vi>)
  n227 = control-ref of="量程下拉列表"() -> (w15:refnum<vi>)
  n228 = control-ref of="备用系数"() -> (w10:refnum<vi>)
  n229 = control-ref of="公式"() -> (w12:refnum<vi>)
  n230 = Obtain Queue(name (unnamed)="TP" ("名称（未命名）"), element data type=cluster{"命令":string, "data":variant} {"命令"="", "data"=variant}) -> (queue out=w17:refnum<queue>, error out=w18:errorcluster)  [unwired: 3 in, 1 out]
  n231 = while {
    tunnel: w17 -> [w461]
    tunnel: w18 -> [_]
    shift-right: [w459] -> _
    shift-left: enum16{"总磷", "总氮"}."总磷" ("枚举") -> [w460]
    stop <- FALSE stop-if-true
    n232 = Get Queue Status(queue=w461) -> (queue out=w456:refnum<queue>, # elements in queue=w455:i32)  [unwired: 2 in, 6 out]
    n233 = Wait (ms)(milliseconds to wait=u32 1000 ("等待时间（毫秒）")) -> ()  [unwired: 1 out]
    n234 = case shown="0" w455 {
      tunnel: w460 -> [w464 w484]
      tunnel: [w464 w483] -> w459
      tunnel: w456 -> [_ w482]
      frame Default {
      }
      frame 0 {
        # "试剂填充 172 \n管路清洗108\n氨氮92\n总磷131\n总磷海水147\n总氮76\n总氮海水92"
        n235 = case shown="\"总氮\", 默认" w484 {
          selector: w484 -> [w488 w490]
          tunnel: [w489 w491] -> w474
          tunnel: [w488 w490] -> w473
          frame "总氮", Default {
            w489 = u16 2 items=["总磷"=1, "总氮"=2] ("站号")
          }
          frame "总磷" {
            w491 = u16 1 items=["总磷"=1, "氨氮"=3] ("站号")
          }
        }
        n236 = global read "VAR总磷总氮全局变量.vi" "状态告警区"() -> (w465:T4)
        n237 = Unbundle By Name(w465) -> ("系统时间"=w472:timestamp)
        n238 = Get Date/Time In Seconds() -> (seconds since 1Jan1904=w471:timestamp)
        n239 = Bundle By Name(cluster=cluster{"命令":string, "data":variant} {"命令"="", "data"=variant} ("元素"), "命令"="读状态告警区", "data"=w474) -> (w480:cluster{"命令":string, "data":variant})
        n240 = Subtract(x=w471, y=w472) -> (x-y=w470:dbl)
        n241 = Bundle By Name(cluster=cluster{"命令":string, "data":variant} {"命令"="", "data"=variant} ("元素"), "命令"="读测量数据区", "data"=w474) -> (w477:cluster{"命令":string, "data":variant})
        n242 = Enqueue Element(queue=w482, element=w480) -> (queue out=w475:refnum<queue>)  [unwired: 2 in, 2 out]
        n243 = Absolute Value(x=w470) -> (abs(x)=w469:dbl)
        n244 = Enqueue Element(queue=w475, element=w477) -> (queue out=w466:refnum<queue>)  [unwired: 2 in, 2 out]
        n245 = Greater Or Equal?(x=w469, y=120.0) -> (x >= y?=w467:bool)
        n246 = case shown="真" w467 {
          tunnel: w466 -> [_ w486]
          frame False {
          }
          frame True {
            n247 = call "总磷总氮启动命令.vi"("参数"=T19 {"站号"=3, "量程切换"=enum."AUTO", "控制命令"=enum."校时", "模式设置"=enum."待机", "测量间隔"=0}) -> ("启动命令"=w485:cluster{"命令":string, "data":variant})  [unwired: 10 in]
            n248 = Enqueue Element(queue=w486, element=w485) -> ()  [unwired: 2 in, 3 out]
          }
        }
        n249 = Increment(x=w473) -> (x+1=w483:enum16{"总磷", "总氮"})
      }
    }
    n250 = global read "总磷总氮断电保存全局变量.vi" "流程路径"() -> (w458:path)
    n251 = global read "总磷总氮断电保存全局变量.vi" "VISA Resource"() -> (→"字符串 2":refnum<visa-resource-name>)
    n252 = local write "流程路径"(w458) -> ()
  }
  n253 = while {
    tunnel: w17 -> [w498]
    tunnel: w15 -> [w497]
    tunnel: w14 -> [w496]
    tunnel: w13 -> [w495]
    tunnel: w12 -> [w494]
    tunnel: w11 -> [w493]
    tunnel: w10 -> [w492]
    tunnel: w5 -> [_]
    stop <- FALSE stop-if-true
    n254 = event shown="[7] \"曲线模型\": 值改变" {
      selector: _ -> [_ _ _ _ _ _ _ _ _ _ _ _ _ _ _ _ _ _ _ _ _ _ _ _ _]
      dyn-events: _ -> [_ _ _ _ _ _ _ _ _ _ _ _ _ _ _ _ _ _ _ _ _ _ _ _ _]
      timeout: _ -> [_ _ _ _ _ _ _ _ _ _ _ _ _ _ _ _ _ _ _ _ _ _ _ _ _]
      tunnel: w498 -> [_ _ w514 w542 _ _ _ _ _ _ _ _ w689 _ w714 w718 _ _ _ _ _ _ _ _ _]
      tunnel: w497 -> [_ _ _ _ _ _ _ _ _ _ _ _ _ _ _ _ _ _ _ w734 _ w777 w786 w794 w805]
      tunnel: w496 -> [_ _ _ _ _ _ _ _ _ _ _ _ _ _ _ _ _ _ _ w732 _ w775 w788 w800 w811]
      tunnel: w495 -> [_ _ _ _ _ _ _ _ _ _ _ _ _ _ _ _ _ _ _ w733 _ w776 w787 w793 w806]
      tunnel: w494 -> [_ _ _ _ _ _ _ _ _ _ _ _ _ _ _ _ _ _ _ w728 _ _ _ _ _]
      tunnel: w493 -> [_ _ _ _ _ _ _ _ _ _ _ _ _ _ _ _ _ _ _ _ _ w771 _ _ _]
      tunnel: w492 -> [_ _ _ _ _ _ _ _ _ _ _ _ _ _ _ _ _ _ _ _ _ _ _ w798 _]
      tunnel: [_ w500 _ _ _ _ _ _ _ _ _ _ _ _ _ _ _ _ _ _ _ _ _ _ _] -> _
      event Timeout {
        n255 = event-data() -> ()  [unwired: 1 in, 3 out]
      }
      event "测量模式下拉列表", "量程下拉列表", "参数下拉列表": Value Change {
        n256 = event-data() -> ()  [unwired: 1 in, 6 out]
        n257 = local read "测量模式下拉列表"() -> (w502:enum16{"水样测量", "零点核查", "跨度核查", "标样核查", "加标回收"})
        n258 = local read "参数下拉列表"() -> (w503:enum16{"总磷", "总氮"})
        n259 = local read "量程下拉列表"() -> (w504:enum16{"低量程", "高量程"})
        n260 = Bundle("参数下拉列表"=w503, "测量模式下拉列表"=w502, "量程下拉列表"=w504) -> (w501:T18)  [unwired: 1 in]
        n261 = property on="曲线模型" class="曲线模型 (严格)"("属性"=w501) -> (error out=w500:errorcluster)  [unwired: 2 in, 1 out]
      }
      event "串口设置": Value Change {
        n262 = event-data() -> ()  [unwired: 1 in, 6 out]
        n263 = global read "总磷总氮断电保存全局变量.vi" "MB通信方式选择"() -> (w505:enum16{"串口", "TCP"})
        n264 = global read "总磷总氮断电保存全局变量.vi" "VISA Resource"() -> (w511:refnum<visa-resource-name>)
        n265 = global read "总磷总氮断电保存全局变量.vi" "PORT"() -> (w509:string)
        n266 = global read "总磷总氮断电保存全局变量.vi" "IP"() -> (w510:string)
        n267 = call "串口配置.vi"("PORT"=w509, "IP"=w510, "MB通信方式选择"=w505, "请选择串口:"=w511) -> ("PORT 2"=w507:string, "IP 2"=w508:string, "确认 2"=w512:bool, "VISA资源名称 2"=w513:refnum<visa-resource-name>, "MB通信方式选择 2"=w506:enum16{"串口", "TCP"})  [unwired: 3 in]
        n268 = case shown="真" w512 {
          tunnel: w513 -> [_ w519]
          tunnel: w514 -> [_ w518]
          tunnel: w508 -> [_ w517]
          tunnel: w507 -> [_ w516]
          tunnel: w506 -> [_ w515]
          frame False {
          }
          frame True {
            n269 = flat-sequence {
              tunnel: w519 -> [w524]
              tunnel: w518 -> [w525]
              tunnel: w517 -> [w523]
              tunnel: w516 -> [w522]
              tunnel: w515 -> [w521]
              frame #0 {
                n270 = global write "总磷总氮断电保存全局变量.vi" "IP"(w523) -> ()
                n271 = global write "总磷总氮断电保存全局变量.vi" "PORT"(w522) -> ()
                n272 = global write "总磷总氮断电保存全局变量.vi" "VISA Resource"(w524) -> ()
                n273 = global write "总磷总氮断电保存全局变量.vi" "MB通信方式选择"(w521) -> ()
                n274 = Flush Queue(queue=w525) -> (queue out=w520:refnum<queue>)  [unwired: 1 in, 2 out]
                n275 = Enqueue Element(queue=w520, element=cluster{"命令":string, "data":variant} {"命令"="启用模块", "data"=variant} ("元素")) -> ()  [unwired: 2 in, 3 out]
              }
              frame #1 {
                n276 = call <vilib>:"Application Directory.vi"() -> ("Application Directory"=w540:path)
                n277 = Build Path(base path=w540, name or relative path="data\\sys.ini" ("名称或相对路径")) -> (appended path=w538:path)
                n278 = call <vilib>:"Open Config Data.vi"("configuration file path"=w538) -> ("error out"=w534:errorcluster, "refnum"=w537:T13)  [unwired: 8 in, 1 out]
                n279 = vi-ref "斯坦道总磷总氮.lvlib:总磷总氮断电保存全局变量.vi"() -> (w536:refnum<vi>)
                n280 = call <userlib>:"Write Panel to INI__ogtk.vi"("error in (no error)"=w534, "VI ref"=w536, "refnum"=w537) -> ("error out"=w533:errorcluster, "refnum out"=w535:T13)  [unwired: 7 in]
                n281 = call <vilib>:"Close Config Data.vi"("error in (no error)"=w533, "refnum"=w535) -> ("error out"=w528:errorcluster, "file path"=w527:path)  [unwired: 8 in]
                n282 = Open/Create/Replace File(file path (use dialog)=w527, error in=w528) -> (refnum out=w531:refnum<file>, error out=w532:errorcluster)  [unwired: 4 in, 1 out]
                n283 = Flush File(refnum=w531, error in=w532) -> (refnum out=w530:refnum<file>, error out=w529:errorcluster)
                n284 = Close File(refnum=w530, error in=w529) -> ()  [unwired: 2 out]
              }
            }
          }
        }
      }
      event "模块启用": Value Change {
        n285 = event-data() -> ("OldVal"=w543:bool)  [unwired: 1 in, 5 out]
        n286 = Flush Queue(queue=w542) -> (queue out=w541:refnum<queue>)  [unwired: 1 in, 2 out]
        n287 = case shown="假" w543 {
          tunnel: w541 -> [w544 w546]
          frame False {
            n288 = Enqueue Element(queue=w544, element=cluster{"命令":string, "data":variant} {"命令"="停用模块", "data"=variant} ("元素")) -> ()  [unwired: 2 in, 3 out]
          }
          frame True {
            n289 = Enqueue Element(queue=w546, element=cluster{"命令":string, "data":variant} {"命令"="启用模块", "data"=variant} ("元素")) -> ()  [unwired: 2 in, 3 out]
          }
        }
      }
      event "流程路径": Value Change {
        n290 = event-data() -> ()  [unwired: 1 in, 6 out]
        n291 = flat-sequence {
          frame #0 {
            n292 = local read "流程路径"() -> (w548:path)
            n293 = global write "总磷总氮断电保存全局变量.vi" "流程路径"(w548) -> ()
          }
          frame #1 {
            n294 = call <vilib>:"Application Directory.vi"() -> ("Application Directory"=w562:path)
            n295 = Build Path(base path=w562, name or relative path="data\\sys.ini" ("名称或相对路径")) -> (appended path=w560:path)
            n296 = call <vilib>:"Open Config Data.vi"("configuration file path"=w560) -> ("error out"=w556:errorcluster, "refnum"=w559:T13)  [unwired: 8 in, 1 out]
            n297 = vi-ref "总磷总氮断电保存全局变量.vi"() -> (w558:refnum<vi>)
            n298 = call <userlib>:"Write Panel to INI__ogtk.vi"("error in (no error)"=w556, "VI ref"=w558, "refnum"=w559) -> ("error out"=w555:errorcluster, "refnum out"=w557:T13)  [unwired: 7 in]
            n299 = call <vilib>:"Close Config Data.vi"("error in (no error)"=w555, "refnum"=w557) -> ("error out"=w550:errorcluster, "file path"=w549:path)  [unwired: 8 in]
            n300 = Open/Create/Replace File(file path (use dialog)=w549, error in=w550) -> (refnum out=w553:refnum<file>, error out=w554:errorcluster)  [unwired: 4 in, 1 out]
            n301 = Flush File(refnum=w553, error in=w554) -> (refnum out=w552:refnum<file>, error out=w551:errorcluster)
            n302 = Close File(refnum=w552, error in=w551) -> ()  [unwired: 2 out]
          }
        }
      }
      event "公式一键写入": Value Change {
        n303 = event-data() -> ()  [unwired: 1 in, 6 out]
        n304 = local read "公式"() -> (w563:cluster{"X^2":dbl, "X":dbl, "b":dbl})
        n305 = call "公式复合写入.vi"("公式"=w563) -> ()  [unwired: 11 in]
      }
      event "备用系数一键写入": Value Change {
        n306 = event-data() -> ()  [unwired: 1 in, 6 out]
        n307 = local read "备用系数"() -> (w564:T2)
        n308 = call "量程参数复合参数写入.vi"("备用系数"=w564) -> ()  [unwired: 11 in]
      }
      event "曲线模型": Value Change {
        n309 = event-data() -> ()  [unwired: 1 in, 6 out]
        n310 = Unbundle By Name("曲线模型") -> ("X^2"=w568:dbl, "X"=w567:dbl, "B"=w566:dbl)
        n311 = local read "公式"() -> (w570:cluster{"X^2":dbl, "X":dbl, "b":dbl})
        n312 = Bundle By Name(cluster=w570, "X^2"=w568, "X"=w567, "b"=w566) -> (w565:cluster{"X^2":dbl, "X":dbl, "b":dbl})
        n313 = local write "公式"(w565) -> ()
      }
      event "质控参数设置": Value Change {
        n314 = event-data() -> ()  [unwired: 1 in, 6 out]
        n315 = global read "总磷总氮断电保存全局变量.vi" "质控参数设置"() -> (w571:T20)
        n316 = call "总磷总氮质控参数设置.vi"("质控参数设置"=w571) -> ("输出簇"=w572:T21)  [unwired: 10 in]
        n317 = Unbundle By Name(w572) -> ("确定"=w573:bool)
        n318 = case shown="真" w573 {
          tunnel: w572 -> [_ w575]
          tunnel: w571 -> [_ w574]
          frame False {
          }
          frame True {
            n319 = flat-sequence {
              tunnel: w575 -> [w586]
              tunnel: w574 -> [w585]
              frame #0 {
                n320 = Unbundle By Name(w586) -> ("总磷跨度值"=w584:dbl, "总磷零点标准液浓度"=w583:dbl, "总磷跨度标准液浓度"=w582:dbl, "总磷标准液标准浓度"=w581:dbl, "总氮跨度值"=w580:dbl, "总氮零点标准液浓度"=w579:dbl, "总氮跨度标准液浓度"=w578:dbl, "总氮标准液标准浓度"=w577:dbl)
                n321 = Bundle By Name(cluster=w585, "总磷跨度值"=w584, "总磷零点标准液浓度"=w583, "总磷跨度标准液浓度"=w582, "总磷标准液标准浓度"=w581, "总氮跨度值"=w580, "总氮零点标准液浓度"=w579, "总氮跨度标准液浓度"=w578, "总氮标准液标准浓度"=w577) -> (w576:T20)
                n322 = global write "总磷总氮断电保存全局变量.vi" "质控参数设置"(w576) -> ()
              }
              frame #1 {
                n323 = call <vilib>:"Application Directory.vi"() -> ("Application Directory"=w600:path)
                n324 = Build Path(base path=w600, name or relative path="data\\sys.ini" ("名称或相对路径")) -> (appended path=w598:path)
                n325 = call <vilib>:"Open Config Data.vi"("configuration file path"=w598) -> ("error out"=w594:errorcluster, "refnum"=w597:T13)  [unwired: 8 in, 1 out]
                n326 = vi-ref "总磷总氮断电保存全局变量.vi"() -> (w596:refnum<vi>)
                n327 = call <userlib>:"Write Panel to INI__ogtk.vi"("error in (no error)"=w594, "VI ref"=w596, "refnum"=w597) -> ("error out"=w593:errorcluster, "refnum out"=w595:T13)  [unwired: 7 in]
                n328 = call <vilib>:"Close Config Data.vi"("error in (no error)"=w593, "refnum"=w595) -> ("error out"=w588:errorcluster, "file path"=w587:path)  [unwired: 8 in]
                n329 = Open/Create/Replace File(file path (use dialog)=w587, error in=w588) -> (refnum out=w591:refnum<file>, error out=w592:errorcluster)  [unwired: 4 in, 1 out]
                n330 = Flush File(refnum=w591, error in=w592) -> (refnum out=w590:refnum<file>, error out=w589:errorcluster)
                n331 = Close File(refnum=w590, error in=w589) -> ()  [unwired: 2 out]
              }
            }
          }
        }
      }
      event "总氮参数设置": Value Change {
        n332 = event-data() -> ()  [unwired: 1 in, 6 out]
        n333 = global read "总磷总氮断电保存全局变量.vi" "总氮仪器参数"() -> (w602:T22)
        n334 = call "仪器参数设置.vi"("氨氮仪器参数"=w602) -> ("仪器参数设置输出"=w601:T23)  [unwired: 10 in]
        n335 = Unbundle By Name(w601) -> ("确定"=w603:bool)
        n336 = case shown="真" w603 {
          tunnel: w601 -> [_ w605]
          tunnel: w602 -> [_ w604]
          frame False {
          }
          frame True {
            n337 = flat-sequence {
              tunnel: w605 -> [w621]
              tunnel: w604 -> [w620]
              frame #0 {
                n338 = Unbundle By Name(w621) -> ("测量量程"=w619:dbl, "测量精度"=w618:dbl, "测量间隔"=w617:dbl, "消解温度"=w616:dbl, "消解时长"=w615:dbl, "空白校准时间"=w614:timestamp, "曲线截距"=w613:dbl, "曲线斜率"=w612:dbl, "测量检出限"=w610:dbl, "测量信号值"=w609:dbl, "线性相关系数"=w608:dbl, "二次多项式系数"=w607:dbl, "标样校准时间"=w606:timestamp)
                n339 = Bundle By Name(cluster=w620, "测量量程"=w619, "测量精度"=w618, "测量间隔"=w617, "消解温度"=w616, "消解时长"=w615, "空白校准时间"=w614, "曲线截距"=w613, "曲线斜率"=w612, "测量检出限"=w610, "测量信号值"=w609, "线性相关系数"=w608, "二次多项式系数"=w607, "标样校准时间"=w606) -> (w611:T22)
                n340 = global write "总磷总氮断电保存全局变量.vi" "总氮仪器参数"(w611) -> ()
              }
              frame #1 {
                n341 = call <vilib>:"Application Directory.vi"() -> ("Application Directory"=w635:path)
                n342 = Build Path(base path=w635, name or relative path="data\\sys.ini" ("名称或相对路径")) -> (appended path=w633:path)
                n343 = call <vilib>:"Open Config Data.vi"("configuration file path"=w633) -> ("error out"=w629:errorcluster, "refnum"=w632:T13)  [unwired: 8 in, 1 out]
                n344 = vi-ref "总磷总氮断电保存全局变量.vi"() -> (w631:refnum<vi>)
                n345 = call <userlib>:"Write Panel to INI__ogtk.vi"("error in (no error)"=w629, "VI ref"=w631, "refnum"=w632) -> ("error out"=w628:errorcluster, "refnum out"=w630:T13)  [unwired: 7 in]
                n346 = call <vilib>:"Close Config Data.vi"("error in (no error)"=w628, "refnum"=w630) -> ("error out"=w623:errorcluster, "file path"=w622:path)  [unwired: 8 in]
                n347 = Open/Create/Replace File(file path (use dialog)=w622, error in=w623) -> (refnum out=w626:refnum<file>, error out=w627:errorcluster)  [unwired: 4 in, 1 out]
                n348 = Flush File(refnum=w626, error in=w627) -> (refnum out=w625:refnum<file>, error out=w624:errorcluster)
                n349 = Close File(refnum=w625, error in=w624) -> ()  [unwired: 2 out]
              }
            }
          }
        }
      }
      event "总磷参数设置": Value Change {
        n350 = event-data() -> ()  [unwired: 1 in, 6 out]
        n351 = global read "总磷总氮断电保存全局变量.vi" "总磷仪器参数"() -> (w637:T22)
        n352 = call "仪器参数设置.vi"("氨氮仪器参数"=w637) -> ("仪器参数设置输出"=w636:T23)  [unwired: 10 in]
        n353 = Unbundle By Name(w636) -> ("确定"=w638:bool)
        n354 = case shown="真" w638 {
          tunnel: w636 -> [_ w640]
          tunnel: w637 -> [_ w639]
          frame False {
          }
          frame True {
            n355 = flat-sequence {
              tunnel: w640 -> [w656]
              tunnel: w639 -> [w655]
              frame #0 {
                n356 = Unbundle By Name(w656) -> ("测量量程"=w654:dbl, "测量精度"=w653:dbl, "测量间隔"=w652:dbl, "消解温度"=w651:dbl, "消解时长"=w650:dbl, "空白校准时间"=w649:timestamp, "曲线截距"=w648:dbl, "曲线斜率"=w647:dbl, "测量检出限"=w645:dbl, "测量信号值"=w644:dbl, "线性相关系数"=w643:dbl, "二次多项式系数"=w642:dbl, "标样校准时间"=w641:timestamp)
                n357 = Bundle By Name(cluster=w655, "测量量程"=w654, "测量精度"=w653, "测量间隔"=w652, "消解温度"=w651, "消解时长"=w650, "空白校准时间"=w649, "曲线截距"=w648, "曲线斜率"=w647, "测量检出限"=w645, "测量信号值"=w644, "线性相关系数"=w643, "二次多项式系数"=w642, "标样校准时间"=w641) -> (w646:T22)
                n358 = global write "总磷总氮断电保存全局变量.vi" "总磷仪器参数"(w646) -> ()
              }
              frame #1 {
                n359 = call <vilib>:"Application Directory.vi"() -> ("Application Directory"=w670:path)
                n360 = Build Path(base path=w670, name or relative path="data\\sys.ini" ("名称或相对路径")) -> (appended path=w668:path)
                n361 = call <vilib>:"Open Config Data.vi"("configuration file path"=w668) -> ("error out"=w664:errorcluster, "refnum"=w667:T13)  [unwired: 8 in, 1 out]
                n362 = vi-ref "总磷总氮断电保存全局变量.vi"() -> (w666:refnum<vi>)
                n363 = call <userlib>:"Write Panel to INI__ogtk.vi"("error in (no error)"=w664, "VI ref"=w666, "refnum"=w667) -> ("error out"=w663:errorcluster, "refnum out"=w665:T13)  [unwired: 7 in]
                n364 = call <vilib>:"Close Config Data.vi"("error in (no error)"=w663, "refnum"=w665) -> ("error out"=w658:errorcluster, "file path"=w657:path)  [unwired: 8 in]
                n365 = Open/Create/Replace File(file path (use dialog)=w657, error in=w658) -> (refnum out=w661:refnum<file>, error out=w662:errorcluster)  [unwired: 4 in, 1 out]
                n366 = Flush File(refnum=w661, error in=w662) -> (refnum out=w660:refnum<file>, error out=w659:errorcluster)
                n367 = Close File(refnum=w660, error in=w659) -> ()  [unwired: 2 out]
              }
            }
          }
        }
      }
      event "总磷自动测试量程配置", "总氮自动测试量程配置": Value Change {
        n368 = event-data() -> ()  [unwired: 1 in, 6 out]
        n369 = flat-sequence {
          frame #0 {
            n370 = global write "总磷总氮断电保存全局变量.vi" "总氮自动测试量程配置"("总氮自动测试量程配置") -> ()
            n371 = global write "总磷总氮断电保存全局变量.vi" "总磷自动测试量程配置"("总磷自动测试量程配置") -> ()
          }
          frame #1 {
            n372 = call <vilib>:"Application Directory.vi"() -> ("Application Directory"=w686:path)
            n373 = Build Path(base path=w686, name or relative path="data\\sys.ini" ("名称或相对路径")) -> (appended path=w684:path)
            n374 = call <vilib>:"Open Config Data.vi"("configuration file path"=w684) -> ("error out"=w680:errorcluster, "refnum"=w683:T13)  [unwired: 8 in, 1 out]
            n375 = vi-ref "总磷总氮断电保存全局变量.vi"() -> (w682:refnum<vi>)
            n376 = call <userlib>:"Write Panel to INI__ogtk.vi"("error in (no error)"=w680, "VI ref"=w682, "refnum"=w683) -> ("error out"=w679:errorcluster, "refnum out"=w681:T13)  [unwired: 7 in]
            n377 = call <vilib>:"Close Config Data.vi"("error in (no error)"=w679, "refnum"=w681) -> ("error out"=w674:errorcluster, "file path"=w673:path)  [unwired: 8 in]
            n378 = Open/Create/Replace File(file path (use dialog)=w673, error in=w674) -> (refnum out=w677:refnum<file>, error out=w678:errorcluster)  [unwired: 4 in, 1 out]
            n379 = Flush File(refnum=w677, error in=w678) -> (refnum out=w676:refnum<file>, error out=w675:errorcluster)
            n380 = Close File(refnum=w676, error in=w675) -> ()  [unwired: 2 out]
          }
        }
      }
      event "手动启动": Value Change {
        n381 = event-data() -> ()  [unwired: 1 in, 6 out]
        n382 = call "总磷总氮启动参数对话框.vi"() -> ("确认"=w687:bool, "元素"=w688:cluster{"命令":string, "data":variant})  [unwired: 10 in]
        n383 = case shown="真" w687 {
          tunnel: w689 -> [_ w691]
          tunnel: w688 -> [_ w690]
          frame False {
          }
          frame True {
            n384 = Enqueue Element(queue=w691, element=w690) -> ()  [unwired: 2 in, 3 out]
          }
        }
      }
      event "定时启动": Mouse Down {
        n385 = event-data() -> ()  [unwired: 1 in, 6 out]
        n386 = flat-sequence {
          frame #0 {
            n387 = global read "总磷总氮断电保存全局变量.vi" "定时控制"() -> (w693:T6)
            n388 = call "总磷总氮周期设置.vi"("定时控制输入"=w693) -> ("定时控制输出"=w692:T24)  [unwired: 10 in]
            n389 = global write "总磷总氮断电保存全局变量.vi" "定时控制"(w692) -> ()
          }
          frame #1 {
            n390 = call <vilib>:"Application Directory.vi"() -> ("Application Directory"=w707:path)
            n391 = Build Path(base path=w707, name or relative path="data\\sys.ini" ("名称或相对路径")) -> (appended path=w705:path)
            n392 = call <vilib>:"Open Config Data.vi"("configuration file path"=w705) -> ("error out"=w701:errorcluster, "refnum"=w704:T13)  [unwired: 8 in, 1 out]
            n393 = vi-ref "总磷总氮断电保存全局变量.vi"() -> (w703:refnum<vi>)
            n394 = call <userlib>:"Write Panel to INI__ogtk.vi"("error in (no error)"=w701, "VI ref"=w703, "refnum"=w704) -> ("error out"=w700:errorcluster, "refnum out"=w702:T13)  [unwired: 7 in]
            n395 = call <vilib>:"Close Config Data.vi"("error in (no error)"=w700, "refnum"=w702) -> ("error out"=w695:errorcluster, "file path"=w694:path)  [unwired: 8 in]
            n396 = Open/Create/Replace File(file path (use dialog)=w694, error in=w695) -> (refnum out=w698:refnum<file>, error out=w699:errorcluster)  [unwired: 4 in, 1 out]
            n397 = Flush File(refnum=w698, error in=w699) -> (refnum out=w697:refnum<file>, error out=w696:errorcluster)
            n398 = Close File(refnum=w697, error in=w696) -> ()  [unwired: 2 out]
          }
        }
      }
      event "单步测试": Value Change {
        w709 = u16 1 items=["总磷"=1, "氨氮"=3] ("站号")
        n399 = event-data() -> ()  [unwired: 1 in, 6 out]
        n400 = Bundle("站号"=w709, "总磷氨氮调试"="总磷氨氮调试") -> (w708:cluster{"站号":u16, "总磷氨氮调试":u16[]})  [unwired: 1 in]
        n401 = Bundle By Name(cluster=cluster{"命令":string, "data":variant} {"命令"="", "data"=variant} ("元素"), "命令"="debug", "data"=w708) -> (w711:cluster{"命令":string, "data":variant})
        n402 = Enqueue Element(queue=w714, element=w711) -> ()  [unwired: 2 in, 3 out]
      }
      event "停止": Value Change {
        n403 = event-data() -> ()  [unwired: 1 in, 6 out]
        n404 = Enqueue Element(queue=w718, element=cluster{"命令":string, "data":variant} {"命令"="启动", "data"=variant(cluster{"站号":u16, "控制命令输出":u16[]} {"站号"=1, "控制命令输出"=[2816]})} ("元素")) -> (queue out=w715:refnum<queue>)  [unwired: 2 in, 2 out]
        n405 = Enqueue Element(queue=w715, element=cluster{"命令":string, "data":variant} {"命令"="启动", "data"=variant(cluster{"站号":u16, "控制命令输出":u16[]} {"站号"=2, "控制命令输出"=[2816]})} ("元素")) -> ()  [unwired: 2 in, 3 out]
      }
      event "设置": Value Change {
        n406 = event-data() -> ()  [unwired: 1 in, 6 out]
        n407 = property on="窗格" class="Pane"("Origin"=T10 {"Horizontal"=0, "Vertical"=628} ("原点")) -> ()  [unwired: 2 in, 2 out]
      }
      event "返回": Value Change {
        n408 = event-data() -> ()  [unwired: 1 in, 6 out]
        n409 = property on="窗格" class="Pane"("Origin"=T10 {"Horizontal"=0, "Vertical"=0} ("原点")) -> ()  [unwired: 2 in, 2 out]
      }
      event "公式.X^2", "公式.X", "公式.b", "量程切换阈值.阈值", "量程切换阈值.标液浓度", "备用系数.量程上限", "备用系数.量程下限", "备用系数.检出限", "备用系数.精度": Mouse Down {
        n410 = event-data() -> ("CtlRef"=w724:refnum<vi>)  [unwired: 1 in, 5 out]
        n411 = property class="DigNum (严格)"(reference=w724) -> (reference out=w722:refnum<vi>, "Value"=w723:dbl)  [unwired: 1 in, 1 out]
        n412 = call "数字键盘.vi"("OldNumber"=w723) -> ("NewNumber"=w721:dbl)
        n413 = property class="DigNum (严格)"(reference=w722, "Val(Sgnl)"=w721) -> ()  [unwired: 1 in, 2 out]
      }
      event "读公式": Value Change {
        n414 = event-data() -> ()  [unwired: 1 in, 6 out]
        n415 = property class="Enum (严格)"(reference=w732) -> ("Value"=w731:enum16{"总磷", "总氮"})  [unwired: 1 in, 2 out]
        n416 = property class="Enum (严格)"(reference=w733) -> ("Value"=w730:enum16{"水样测量", "零点核查", "跨度核查", "标样核查", "加标回收"})  [unwired: 1 in, 2 out]
        n417 = property class="Enum (严格)"(reference=w734) -> ("Value"=w729:enum16{"低量程", "高量程"})  [unwired: 1 in, 2 out]
        n418 = call "总磷总氮公式读取.vi"("量程"=w729, "测量模式"=w730, "测量参数"=w731) -> ("error out"=w726:errorcluster, "公式"=w727:cluster{"X^2":dbl, "X":dbl, "b":dbl})  [unwired: 7 in]
        n419 = property class="Clust (严格)"(reference=w728, "Value"=w727) -> ()  [unwired: 1 in, 2 out]
        n420 = case shown="错误" w726 {
          tunnel: ["读取成功" ("消息") "读取失败" ("消息")] -> w725
          frame No Error {
          }
          frame Error {
          }
        }
        n421 = One Button Dialog(message=w725) -> ()  [unwired: 1 in, 1 out]
      }
      event "写公式": Value Change {
        n422 = event-data() -> ()  [unwired: 1 in, 6 out]
        n423 = call "总磷总氮公式写入.vi"("公式"="公式", "量程"="量程下拉列表", "测量模式"="测量模式下拉列表", "测量参数"="参数下拉列表") -> ("error out"=w741:errorcluster)  [unwired: 7 in]
        n424 = case shown="无错误" w741 {
          tunnel: ["写入成功" ("消息") "写入失败" ("消息")] -> w742
          tunnel: "公式" -> [w751 _]
          tunnel: "测量模式下拉列表" -> [w749 _]
          tunnel: "量程下拉列表" -> [w747 _]
          tunnel: "参数下拉列表" -> [w746 _]
          frame No Error {
            n425 = Equal?(x=w747, y=enum16{"低量程", "高量程"}."低量程" ("量程下拉列表")) -> (x = y?=w744:bool)
            n426 = Equal?(x=w749, y=enum16{"水样测量", "零点核查", "跨度核查", "标样核查", "加标回收"}."水样测量" ("测量模式下拉列表")) -> (x = y?=w745:bool)
            n427 = And(x=w745, y=w744) -> (x .and. y?=w743:bool)
            n428 = case shown="真" w743 {
              tunnel: w751 -> [_ w754]
              tunnel: w746 -> [_ w753]
              frame False {
              }
              frame True {
                n429 = case shown="\"总磷\", 默认" w753 {
                  tunnel: w754 -> [w755 w761]
                  frame "总磷", Default {
                    n430 = Unbundle By Name(w755) -> ("X^2"=w758:dbl, "X"=w757:dbl, "b"=w756:dbl)
                    n431 = global read "总磷总氮断电保存全局变量.vi" "总磷仪器参数"() -> (w759:T22)
                    n432 = Bundle By Name(cluster=w759, "曲线截距"=w756, "曲线斜率"=w757, "二次多项式系数"=w758) -> (w760:T22)
                    n433 = global write "总磷总氮断电保存全局变量.vi" "总磷仪器参数"(w760) -> ()
                  }
                  frame "总氮" {
                    n434 = Unbundle By Name(w761) -> ("X^2"=w764:dbl, "X"=w763:dbl, "b"=w762:dbl)
                    n435 = global read "总磷总氮断电保存全局变量.vi" "总氮仪器参数"() -> (w765:T22)
                    n436 = Bundle By Name(cluster=w765, "曲线截距"=w762, "曲线斜率"=w763, "二次多项式系数"=w764) -> (w766:T22)
                    n437 = global write "总磷总氮断电保存全局变量.vi" "总氮仪器参数"(w766) -> ()
                  }
                }
              }
            }
          }
          frame Error {
          }
        }
        n438 = One Button Dialog(message=w742) -> ()  [unwired: 1 in, 1 out]
      }
      event "量程切换阈值读取": Value Change {
        n439 = event-data() -> ()  [unwired: 1 in, 6 out]
        n440 = property class="Enum (严格)"(reference=w775) -> ("Value"=w774:enum16{"总磷", "总氮"})  [unwired: 1 in, 2 out]
        n441 = property class="Enum (严格)"(reference=w776) -> ("Value"=w773:enum16{"水样测量", "零点核查", "跨度核查", "标样核查", "加标回收"})  [unwired: 1 in, 2 out]
        n442 = property class="Enum (严格)"(reference=w777) -> ("Value"=w772:enum16{"低量程", "高量程"})  [unwired: 1 in, 2 out]
        n443 = call "总磷总氮量程读取.vi"("量程"=w772, "测量模式"=w773, "测量参数"=w774) -> ("error out"=w768:errorcluster, "量程切换阈值"=w770:cluster{"阈值":dbl, "标液浓度":dbl})  [unwired: 7 in]
        n444 = property class="Clust (严格)"(reference=w771, "Value"=w770) -> ()  [unwired: 1 in, 2 out]
        n445 = case shown="错误" w768 {
          tunnel: ["读取成功" ("消息") "读取失败" ("消息")] -> w769
          frame No Error {
          }
          frame Error {
          }
        }
        n446 = One Button Dialog(message=w769) -> ()  [unwired: 1 in, 1 out]
      }
      event "量程切换阈值写入": Value Change {
        n447 = event-data() -> ()  [unwired: 1 in, 6 out]
        n448 = property class="Enum (严格)"(reference=w788) -> ("Value"=w785:enum16{"总磷", "总氮"})  [unwired: 1 in, 2 out]
        n449 = property class="Enum (严格)"(reference=w787) -> ("Value"=w784:enum16{"水样测量", "零点核查", "跨度核查", "标样核查", "加标回收"})  [unwired: 1 in, 2 out]
        n450 = property class="Enum (严格)"(reference=w786) -> ("Value"=w783:enum16{"低量程", "高量程"})  [unwired: 1 in, 2 out]
        n451 = call "总磷总氮量程写入.vi"("量程切换阈值"="量程切换阈值", "量程"=w783, "测量模式"=w784, "测量参数"=w785) -> ("error out"=w780:errorcluster)  [unwired: 7 in]
        n452 = case shown="无错误" w780 {
          tunnel: ["写入成功" ("消息") "写入失败" ("消息")] -> w781
          frame No Error {
          }
          frame Error {
          }
        }
        n453 = One Button Dialog(message=w781) -> ()  [unwired: 1 in, 1 out]
      }
      event "备用系数读取": Value Change {
        n454 = event-data() -> ()  [unwired: 1 in, 6 out]
        n455 = property class="Enum (严格)"(reference=w800) -> ("Value"=w799:enum16{"总磷", "总氮"})  [unwired: 1 in, 2 out]
        n456 = property class="Enum (严格)"(reference=w793) -> ("Value"=w792:enum16{"水样测量", "零点核查", "跨度核查", "标样核查", "加标回收"})  [unwired: 1 in, 2 out]
        n457 = property class="Enum (严格)"(reference=w794) -> ("Value"=w791:enum16{"低量程", "高量程"})  [unwired: 1 in, 2 out]
        n458 = call "总磷总氮备用系数读取.vi"("量程"=w791, "测量模式"=w792, "测量参数"=w799) -> ("error out"=w795:errorcluster, "备用系数"=w797:T2)  [unwired: 7 in]
        n459 = property class="Clust (严格)"(reference=w798, "Value"=w797) -> ()  [unwired: 1 in, 2 out]
        n460 = case shown="错误" w795 {
          tunnel: ["读取成功" ("消息") "读取失败" ("消息")] -> w796
          frame No Error {
          }
          frame Error {
          }
        }
        n461 = One Button Dialog(message=w796) -> ()  [unwired: 1 in, 1 out]
      }
      event "备用系数写入": Value Change {
        n462 = event-data() -> ()  [unwired: 1 in, 6 out]
        n463 = property class="Enum (严格)"(reference=w811) -> ("Value"=w810:enum16{"总磷", "总氮"})  [unwired: 1 in, 2 out]
        n464 = property class="Enum (严格)"(reference=w806) -> ("Value"=w804:enum16{"水样测量", "零点核查", "跨度核查", "标样核查", "加标回收"})  [unwired: 1 in, 2 out]
        n465 = property class="Enum (严格)"(reference=w805) -> ("Value"=w803:enum16{"低量程", "高量程"})  [unwired: 1 in, 2 out]
        n466 = call "总磷总氮备用系数写入.vi"("备用系数"="备用系数", "量程"=w803, "测量模式"=w804, "测量参数"=w810) -> ("error out"=w807:errorcluster)  [unwired: 7 in]
        n467 = case shown="无错误" w807 {
          tunnel: ["写入成功" ("消息") "写入失败" ("消息")] -> w808
          frame No Error {
          }
          frame Error {
          }
        }
        n468 = One Button Dialog(message=w808) -> ()  [unwired: 1 in, 1 out]
      }
    }
  }
